vi "WS1050 36 DUT CV Curve Ver1.2.vi"() -> ()   [LabVIEW 2012]
uses:
  WS_VCAP Driver 029/Source/WSVCAP Shell/Type Defs/WSVCAP SHL I2C DUT Mask Mode Enum.ctl
panel:
  out "VISA resource name out":refnum<visa-resource-name>="GPIB0::3::INSTR"
  out "error out 2":errorcluster={"status"=TRUE, "code"=-63192, "source"="niLvFpga_Open_PXI-7813R.vi"}
  in  "Reg1_Bit Cntrl":string[](array[string])=["01", "02", "04", "08", "10", "20", "40", "80", "03", "06", "0C", "D8", "33", "66", "CC", "07", "0E", "1C", "38", "70", "E0", "0F", "1E", "3C", "78", "F0", "1F", "3E", "7C", "F8", "3F", "7E", "FC", "7F", "FE", "FD", "FB", "F7", "EF", "DF", "BF", "7F", "FC", "F9", "F3", "E7", "CF", "9F", "3F", "F8", "F1", "E3", "C7", "8F", "1F", "F0", "E1", "C3", "87", "0F", "E0", "C1", "83", "07", "C0", "81", "03", "AA", "55", "00"]
  out "date string":string="5/19/2014"
  out "PS1 Out":refnum<visa-resource-name>
  out "Ke2000 Out":refnum<visa-resource-name>="GPIB0::9::INSTR"
  in  "Tab Control":T1(tab)
  in  "Board#":string="BRD5"
  in  "Serial Number":string[][](table)=[["DUT", "SN"], ["DUT1", "1"], ["DUT2", "2"], ["DUT3", "3"], ["DUT4", "4"], ["DUT5", "5"], ["DUT6", "6"], ["DUT7", "7"], ["DUT8", "8"], ["DUT9", "9"], ["DUT10", "10"], ["DUT11", "11"], ["DUT12", "12"], ["DUT13", "13"], ["DUT14", "14"], ["DUT15", "15"], ["DUT16", "16"], ["DUT17", "17"], ["DUT18", "18"], ["DUT19", "19"], ["DUT20", "20"], ["DUT21", "21"], ["DUT22", "22"], ["DUT23", "23"], ["DUT24", "24"], ["DUT25", "25"], ["DUT26", "26"], ["DUT27", "27"], ["DUT28", "28"], ["DUT29", "29"], ["DUT30", "30"], ["DUT31", "31"], ["DUT32", "32"], ["DUT33", "33"], ["DUT34", "34"], ["DUT35", "35"], ["DUT36", "36"]]
  in  "Wafer#":string="T7-EB"
  in  "File Name":string="CP Sweep_WS1050_T7_EB_25C_BRD4_160706_1"
  in  "TMN DC\\CAP Data Log File Path":path=path "C:/WS1050 36 DUT Data"
  in  "Test Program":string="WS1050 36 DUT CV Curve Ver1.2"
  out "Current Date":string="8/28/2014"
  out "Current Time":string="0950"
  in  "Start Date":string="10/21/2014"
  in  "Start Time":string="1542"
  in  "Comment":string="CP Sweep RT"
  in  "OK Button":bool
  in  "Calibration":bool
  in  "Verify CP":bool
  in  "CP Setting":i32(ring) items=["CP OFF", "CP ON", "CP 35V", "CP 40V", "DVA ON", "DVA OFF", "REG1 ON", "REG1 OFF", "REG2 ON", "REG2 OFF", "REG3 ON", "REG3 OFF"]
  in  "Set VDD":dbl=3.3 format="%.3g"
  in  "Clock Rate (Hz)":dbl=1000000.0 caption="Meas Speed" format="%.1p Hz"
  out "AR  Measurent(Hz)":dbl
  in  "PS1 Source":refnum<visa-resource-name>="GPIB0::5::INSTR"
  in  "Ke2000":refnum<visa-resource-name>="GPIB0::9::INSTR"
  in  "CP to HD/Cycle":i32(ring)=1 items=["CP HDC 35V", "CP HDC 40.25V", "CP HDC 27.5V", "CP HDC 30.5V", "CP HDC 44V"]
  out "Simulate FPGA":bool
  out "Online":bool
  in  "Ke2400":refnum<visa-resource-name>="GPIB0::3::INSTR"
  in  "Initialize AD7747":bool
  in  "DUT Mask Mode":T2=enum."All"
  in  "RFFE Slave Address":u8=7 caption="Slave Address" format="0x%02x"
  out "Activity Log":string="05/19/2014 -- 12:24:35.853::WSVCAP::APP::Application Started\n05/19/2014 -- 12:24:37.606::WSVCAP::WSVCAP SHL::WR I2C-REG:0x0A;MASK:0xFFFFFFFFFFFF;C1 DATA:22:22:22:22:22:22:22:22:22:22:22:22:22:22:22:22;C2 DATA:22:22:22:22:22:22:22:22:22:22:22:22:22:22:22:22;C3 DATA:22:22:22:22:22:22:22:22:22:22:22:22:22:22:22:22\r\n05/19/2014 -- 12:24:37.773::WSVCAP::WSVCAP SHL::WR I2C-ST:0,0,4,1\r\n05/19/2014 -- 12:24:37.903::WSVCAP::WSVCAP SHL::RD I2C-BYTES:4;ADD:0x00;MASK:0xFFFFFFFFFFFF\r\n05/19/2014 -- 12:24:38.045::WSVCAP::WSVCAP SHL::RD I2C:C1 DATA:2:2:2:2:2:2:2:2:2:2:2:2:2:2:2:2|A7:A9:AA:82:82:7F:82:81:82:81:83:82:81:82:82:81|46:36:BB:88:44:A3:E9:2B:32:20:ED:25:BB:3D:68:B|2C:6A:EB:A7:22:56:FE:CC:36:82:D7:B0:3B:48:F9:CC;C2 DATA:2:2:2:2:2:2:2:2:2:2:2:2:2:2:2:2|94:94:94:80:80:80:80:80:81:7E:7E:81:80:7E:80:80|47:33:15:82:62:B:E8:1C:D7:C3:7D:41:7C:B7:4C:2A|C4:B4:AE:8:1E:D1:4E:37:11:C0:6F:63:42:9D:63:B5;C3 DATA:2:2:2:2:2:2:2:2:2:2:2:2:2:2:2:2|95:95:95:81:81:7E:81:80:84:7D:80:83:81:7E:7F:80|AB:C4:14:B5:7B:52:DF:C9:79:5D:5F:30:99:31:1E:F4|6E:5C:F7:A8:C3:EB:7B:EF:33:92:89:77:4D:67:75:DD;STATUS:0:0:4:0\r\n05/19/2014 -- 12:24:38.046::WSVCAP::WSVCAP SHL::WR I2C-REG:0x0A;MASK:0xFFFFFFFFFFFF;C1 DATA:22:22:22:22:22:22:22:22:22:22:22:22:22:22:22:22;C2 DATA:22:22:22:22:22:22:22:22:22:22:22:22:22:22:22:22;C3 DATA:22:22:22:22:22:22:22:22:22:22:22:22:22:22:22:22\r\n05/19/2014 -- 12:24:38.089::WSVCAP::WSVCAP SHL::WR I2C-ST:0,0,4,1\r\n05/19/2014 -- 12:24:38.219::WSVCAP::WSVCAP SHL::RD I2C-BYTES:4;ADD:0x00;MASK:0xFFFFFFFFFFFF\r\n05/19/2014 -- 12:24:38.362::WSVCAP::WSVCAP SHL::RD I2C:C1 DATA:2:2:2:2:2:2:2:2:2:2:2:2:2:2:2:2|A7:AB:AA:82:82:82:83:83:82:82:82:82:7F:82:82:81|4B:32:96:83:3E:61:43:17:25:62:AB:4D:A2:40:2E:5|3C:76:2B:B4:EE:E4:A9:1A:AA:A:26:C7:21:2E:87:5B;C2 DATA:2:2:2:2:2:2:2:2:2:2:2:2:2:2:2:2|94:94:94:80:80:80:80:80:80:7F:80:81:80:80:7F:80|4A:32:19:7D:19:6C:79:46:61:7F:4B:B8:A5:30:F3:14|B4:70:A:8C:9C:DC:43:FA:1E:A:C6:21:A:A9:13:F3;C3 DATA:2:2:2:2:2:2:2:2:2:2:2:2:2:2:2:2|95:97:94:81:80:81:82:81:80:7E:81:84:7F:81:80:80|B2:32:D0:A7:9E:4C:AB:D4:EE:D9:F0:82:B7:91:7:FF|C1:91:B6:3D:D8:E:1B:4F:9F:6A:F1:6C:E7:3F:7:BA;STATUS:0:0:4:0\r\n05/19/2014 -- 12:24:38.364::WSVCAP::WSVCAP SHL::WR I2C-REG:0x0A;MASK:0xFFFFFFFFFFFF;C1 DATA:22:22:22:22:22:22:22:22:22:22:22:22:22:22:22:22;C2 DATA:22:22:22:22:22:22:22:22:22:22:22:22:22:22:22:22;C3 DATA:22:22:22:22:22:22:22:22:22:22:22:22:22:22:22:22\r\n05/19/2014 -- 12:24:38.406::WSVCAP::WSVCAP SHL::WR I2C-ST:0,0,4,1\r\n05/19/2014 -- 12:24:38.536::WSVCAP::WSVCAP SHL::RD I2C-BYTES:4;ADD:0x00;MASK:0xFFFFFFFFFFFF\r\n05/19/2014 -- 12:24:38.678::WSVCAP::WSVCAP SHL::RD I2C:C1 DATA:2:2:2:2:2:2:2:2:2:2:2:2:2:2:2:2|A7:A9:AB:82:82:81:82:82:82:82:82:82:82:82:82:81|46:71:4C:87:43:3D:7F:FC:25:4F:8E:54:97:3E:60:8C|AA:F4:1F:B5:CE:43:1F:36:9:87:9C:78:86:5:B6:8E;C2 DATA:2:2:2:2:2:2:2:2:2:2:2:2:2:2:2:2|94:94:94:80:7F:7F:80:80:80:80:80:81:80:80:80:80|49:36:18:7D:6E:C5:E4:3C:81:2E:41:D3:75:71:E3:72|E8:D3:E6:D1:E0:48:AE:D4:54:D:E8:8E:B4:41:68:4;C3 DATA:2:2:2:2:2:2:2:2:2:2:2:2:2:2:2:2|95:95:95:81:7F:7F:81:81:81:81:81:84:81:81:82:81|B3:F5:90:AB:82:69:7B:93:D0:77:E8:D5:E8:8C:84:E8|B9:AC:EE:2B:B6:71:8F:4A:74:31:56:BB:8A:B7:A0:C8;STATUS:0:0:4:0\r\n05/19/2014 -- 12:24:38.681::WSVCAP::WSVCAP SHL::WR I2C-REG:0x0A;MASK:0xFFFFFFFFFFFF;C1 DATA:22:22:22:22:22:22:22:22:22:22:22:22:22:22:22:22;C2 DATA:22:22:22:22:22:22:22:22:22:22:22:22:22:22:22:22;C3 DATA:22:22:22:22:22:22:22:22:22:22:22:22:22:22:22:22\r\n05/19/2014 -- 12:24:38.723::WSVCAP::WSVCAP SHL::WR I2C-ST:0,0,4,1\r\n05/19/2014 -- 12:24:38.854::WSVCAP::WSVCAP SHL::RD I2C-BYTES:4;ADD:0x00;MASK:0xFFFFFFFFFFFF\r\n05/19/2014 -- 12:24:38.996::WSVCAP::WSVCAP SHL::RD I2C:C1 DATA:2:2:2:2:2:2:2:2:2:2:2:2:2:2:2:2|A7:A9:AA:82:82:7F:83:81:82:81:84:82:7F:82:7F:82|43:FB:E:7F:3C:AD:35:35:26:A2:6C:21:4B:3D:8:6|63:9A:E1:F3:95:32:91:42:90:3C:78:1F:5C:D7:5F:D8;C2 DATA:2:2:2:2:2:2:2:2:2:2:2:2:2:2:2:2|94:94:94:80:80:80:80:80:81:80:7E:81:80:7E:7F:80|48:36:18:7F:5E:3D:69:83:DE:AE:A1:9E:31:AE:BB:96|15:A0:44:17:13:FD:CC:C8:6D:B2:EF:A7:C:C7:3B:F;C3 DATA:2:2:2:2:2:2:2:2:2:2:2:2:2:2:2:2|95:96:94:81:81:7E:82:80:84:80:80:84:7F:7E:7D:82|AD:3B:6D:A9:7C:57:9D:F5:7A:96:23:5C:36:2D:ED:5A|CD:46:DB:3B:C7:BD:70:60:33:B8:B:F7:63:A:51:4D;STATUS:0:0:4:0\r\n05/19/2014 -- 12:24:38.998::WSVCAP::WSVCAP SHL::WR I2C-REG:0x0A;MASK:0xFFFFFFFFFFFF;C1 DATA:22:22:22:22:22:22:22:22:22:22:22:22:22:22:22:22;C2 DATA:22:22:22:22:22:22:22:22:22:22:22:22:22:22:22:22;C3 DATA:22:22:22:22:22:22:22:22:22:22:22:22:22:22:22:22\r\n05/19/2014 -- 12:24:39.040::WSVCAP::WSVCAP SHL::WR I2C-ST:0,0,4,1\r\n05/19/2014 -- 12:24:39.170::WSVCAP::WSVCAP SHL::RD I2C-BYTES:4;ADD:0x00;MASK:0xFFFFFFFFFFFF\r\n05/19/2014 -- 12:24:39.311::WSVCAP::WSVCAP SHL::RD I2C:C1 DATA:2:2:2:2:2:2:2:2:2:2:2:2:2:2:2:2|A7:AA:AB:82:82:81:82:81:82:81:82:82:82:82:7F:82|44:F1:90:87:45:44:C8:2C:2C:F1:FC:1B:94:3B:3C:75|4A:49:95:19:99:73:64:3:23:24:F3:A2:5E:7F:C4:B6;C2 DATA:2:2:2:2:2:2:2:2:2:2:2:2:2:2:2:2|94:94:94:80:80:80:80:7F:80:80:7E:80:80:7E:7F:80|4C:36:17:7D:A8:9F:DE:C7:53:6D:8A:F4:41:A5:C6:E0|90:2E:24:C:D9:22:E4:76:3B:40:1D:53:33:B1:3E:4D;C3 DATA:2:2:2:2:2:2:2:2:2:2:2:2:2:2:2:2|95:97:95:81:81:7F:81:80:80:81:7F:82:81:7E:7D:82|AE:2B:A7:AB:CC:CD:A4:38:FD:17:80:F2:92:2D:45:C4|76:E5:D:B9:AD:B5:BA:8D:28:32:9E:42:B7:20:4A:D9;STATUS:0:0:4:0\r\n05/19/2014 -- 12:24:39.313::WSVCAP::WSVCAP SHL::WR I2C-REG:0x0A;MASK:0xFFFFFFFFFFFF;C1 DATA:22:22:22:22:22:22:22:22:22:22:22:22:22:22:22:22;C2 DATA:22:22:22:22:22:22:22:22:22:22:22:22:22:22:22:22;C3 DATA:22:22:22:22:22:22:22:22:22:22:22:22:22:22:22:22\r\n05/19/2014 -- 12:24:39.355::WSVCAP::WSVCAP SHL::WR I2C-ST:0,0,4,1\r\n05/19/2014 -- 12:24:39.486::WSVCAP::WSVCAP SHL::RD I2C-BYTES:4;ADD:0x00;MASK:0xFFFFFFFFFFFF\r\n05/19/2014 -- 12:24:39.628::WSVCAP::WSVCAP SHL::RD I2C:C1 DATA:2:2:2:2:2:2:2:2:2:2:2:2:2:2:2:2|A7:A9:AA:82:82:82:83:82:82:82:82:82:7F:82:7F:82|47:18:E4:87:3E:E7:6:65:25:92:37:38:A8:3E:89:85|7C:A7:7:2B:A3:7A:EC:EF:89:ED:F4:D3:D8:BC:3A:F5;C2 DATA:2:2:2:2:2:2:2:2:2:2:2:2:2:2:2:2|94:94:94:80:7F:80:80:7F:81:80:7E:80:80:80:81:80|49:37:17:80:76:25:6A:F8:DF:55:97:4D:B8:5B:2B:B1|13:E3:9A:3E:1A:2D:4F:B6:DB:E9:61:FA:8B:D6:9:CC;C3 DATA:2:2:2:2:2:2:2:2:2:2:2:2:2:2:2:2|95:95:95:81:7F:80:82:81:84:80:7F:81:80:81:7F:82|AF:93:3B:AF:5B:11:82:E4:7E:C3:2D:72:9:96:D9:A|DB:96:F2:10:5F:64:9A:C6:98:12:27:7D:10:D3:20:D9;STATUS:0:0:4:0\r\n05/19/2014 -- 12:24:40.132::WSVCAP::WSVCAP SHL::CLOSE\r\n"
  in  "C1 Cap DAC":u8=128 caption="B Data In" format="0x%02x"
  in  "C2 Cap DAC":u8=128 caption="B Data In" format="0x%02x"
  in  "C3 Cap DAC":u8=128 caption="B Data In" format="0x%02x"
  out "IDD Brd(uA)":string
  in  "Control Panel":T3={"Verify Socket"=FALSE, "HD/CYC"=FALSE, "E-CAL"=FALSE, "DVA"=FALSE, "VPI"=TRUE, "VSA"=FALSE, "HS"=FALSE}
  out "Verify Socket":bool
  out "HD/CYC":bool
  out "E-CAL":bool
  out "DVA":bool
  out "VPI":bool
  out "VSA":bool
  out "HS":bool
  in  "Lot#":string="WS1050"
  out "AD7747 Values":string[][](table)
  in  "Freq(Hz)":string="NA"
  in  "Reset P/S":bool
  in  "Test Sequences":i32(ring) items=["C1_C2_C3", "C2_C1_C3", "C3_C2_C1"]
  in  "WS1050/51":bool=TRUE
  in  "CP with DVA ON":i32(ring) items=["CP HDC 35V", "CP HDC 40.25V", "CP HDC 27.5V", "CP HDC 30.5V", "CP HDC 44V"]
  in  "CP Sweep":bool=TRUE
  in  "Serialize":bool
  in  "Start No":i32=1
  in  "VPI Name":string[](array[string])=["All Drivers ON"]
  in  "VPI_Cmd":string[](array[string])=["3B"]
  in  "Temperature":string="25C"
  out "40V_1":string[][](table)
  out "NOM IDD OFF(uA)":string
  out "40V_2":string[][](table)
  out "40V_3":string[][](table)
  out "Previous Time":string="12:20:26 PM"
  out "STATUS":string="Idle...."
  out "Total Delta C2(pF)":string[](array[string])
  out "Total Delta C1(pF)":string[](array[string])
  out "Total Delta C3(pF)":string[](array[string])
  out "RB Reg for HD/Cycle":string[](array[string])
  out "VPI C2":string[][](table)
  out "VPI C3":string[][](table)
  out "NOM IDD ON (uA)":string
  out "IDD_HD/CYC (uA)":string="164.601255E+0"
  in  "stop":bool
  out "IDD Stdby(uA)":string="2.606990E+0"
  out "VPI C1":string[][](table)
  in  "TTF Completed":i32=60
  out "Loop Completed":i32
  out "VSA_V1":string[][](table)
  out "VSA_V2":string[][](table)
  out "VSA_V3":string[][](table)
  in  "VSA Voltage(V)":dbl[](array[numeric])=[-27.0, 0.0, 27.0]
  in  "X Repeat":i32=100
  out "% Delta C_T0":string[][](array[string])
  out "% Delta C":string[][](array[string])
  out "EFuse RB T0":string[](array[string])
  out "Current EFuse Read back":string[](array[string])
  out "EFuse Readback Status":bool[](array[boolean])
  in  "DeltaC Target Setting(pF)":dbl=7.375
  out "error out":errorcluster
  in  "error in (no error)":errorcluster
  in  "Bank 2":i32(ring)=1 items=["C1", "C2", "C3", "D_C1", "D_C2", "D_C3"]
  out "DeltaC Change_1":dbl[][](graph) caption="(Y) Multi Plot 2"
  out "DeltaC Change_2":dbl[][](graph) caption="(Y) Multi Plot 2"
  out "DeltaC Change_3":dbl[][](graph) caption="(Y) Multi Plot 2"
  in  "Debug":bool
  in  "No of Rows\nFrom Spread Sheet":i32
  in  "Plot Delta Cmin":bool=TRUE
  in  "Plot":T4(ring)
  in  "Bank 1":i32(ring) items=["C1", "C2", "C3", "D_C1", "D_C2", "D_C3"]
  in  "Bank 3":i32(ring)=2 items=["C1", "C2", "C3", "D_C1", "D_C2", "D_C3"]
  in  "Col C1":i32=5
  in  "Col C2":i32=6
  in  "Col C3":i32=7
  # "Company:  WiSpry Inc\n20 Fairbanks Ste 198 Irvine CA 92618\n\nAuthor:  Andy V Tran\nCreated:  07/06/2016\nLabVIEW 2012 Pro\nTest Program:  WS1050 36 DUT \nCP Sweep ver1.2\nFPGA: WS_VCAP Driver 029"
  # "Note for CP CV Sweep:\n\n1.  CP will sweep from Low to High to Low\n2.  CP will sweep by banks\n3.  VPI will be checked for CP CV Sweep"
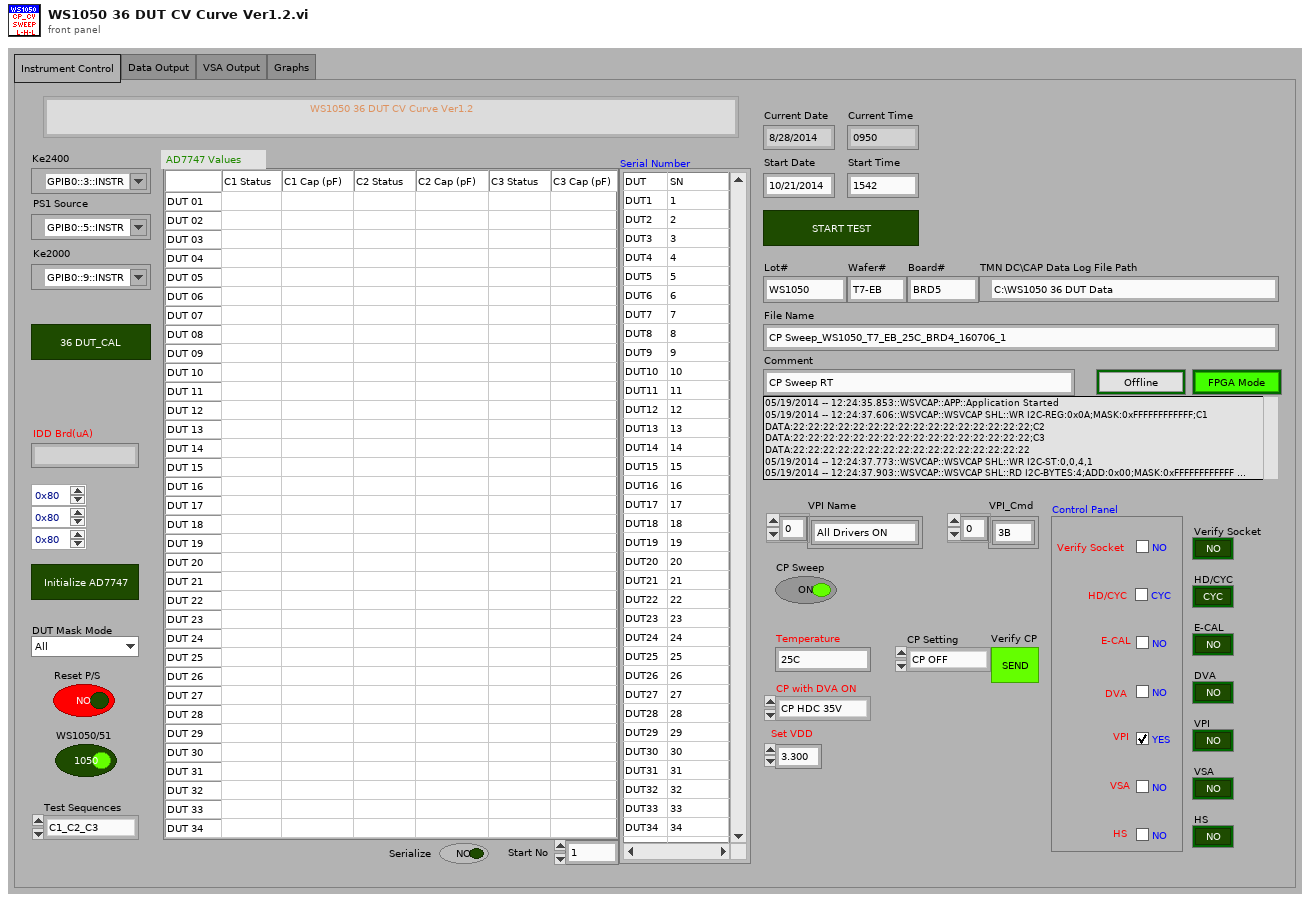
[diagram p1: front panel]
types:
  T1 = enum32{"Instrument Control", "Data Output", "VSA Output", "Graphs"}
  T2 = typedef "WSVCAP SHL I2C DUT Mask Mode Enum.ctl" = enum16{"Custom", "C1", "C2", "C3", "All"}
  T3 = cluster{"Verify Socket":bool, "HD/CYC":bool, "E-CAL":bool, "DVA":bool, "VPI":bool, "VSA":bool, "HS":bool}
  T4 = enum16{"ALL DUTs", "DUT 01", "DUT 02", "DUT 03", "DUT 04", "DUT 05", "DUT 06", "DUT 07", "DUT 08", "DUT 09", "DUT 10", "DUT 11", "DUT 12", "DUT 13", "DUT 14", "DUT 15", "DUT 16", "DUT 17", "DUT 18", "DUT 19", "DUT 20", "DUT 21", "DUT 22", "DUT 23", "DUT 24", "DUT 25", "DUT 26", "DUT 27", "DUT 28", "DUT 29", "DUT 30", "DUT 31", "DUT 32", "DUT 33", "DUT 34", "DUT 35", "DUT 36"}
  T5 = typedef "WSVCAP SHL Core System Cluster.ctl" = cluster{"Settings":T6, "FPGA Resource":tag, "Online":bool, "I2C Wait Ticks":u32, "SPI Wait Ticks":u32, "RFFE Wait Ticks":u32}
  T6 = typedef "WSVCAP SHL I2C Settings Cluster.ctl" = cluster{"FPGA Resource Name":string, "I2C Slave Address":u8, "I2C Clock Rate (Hz)":dbl, "SPI Clock Rate (Hz)":dbl, "RFFE Slave Address":u8, "RFFE Clock Rate (Hz)":dbl, "Simulate FPGA":bool, "C1 Cap DAC Default":u8, "C2 Cap DAC Default":u8, "C3 Cap DAC Default":u8}
  T7 = enum16{"Idle...", "Voltage 1", "Voltage 2", "Voltage 3"}
  T8 = enum16{"Idle...", "Voltage 1", "Voltage 2", "Voltage 3"}[]
  T9 = cluster{"Test Program ":string, "Comment":string, "Data Out":string, "Data Out":string, "Data Out":string, string, "Data Out":string, "Data Out":string, "Data Out":string, "Freq(Hz)":string, "Board#":string}
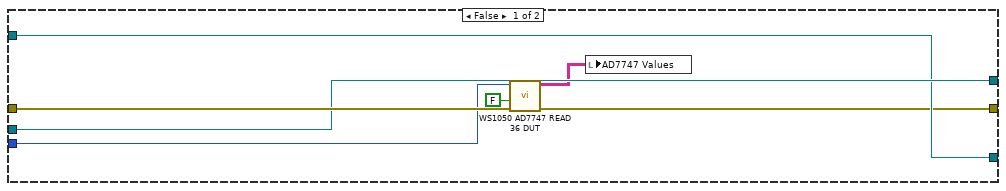
[diagram p9: hidden frame]
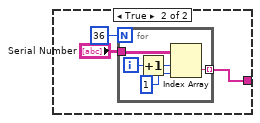
[diagram p10: hidden frame]
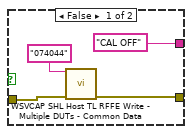
[diagram p11: hidden frame]
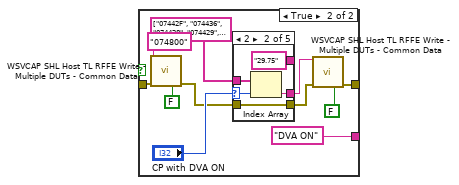
[diagram p12: hidden frame]
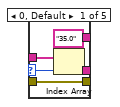
[diagram p13: hidden frame]
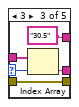
[diagram p14: hidden frame]
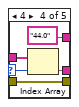
[diagram p15: hidden frame]
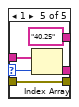
[diagram p16: hidden frame]
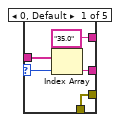
[diagram p17: hidden frame]
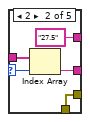
[diagram p18: hidden frame]
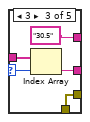
[diagram p19: hidden frame]
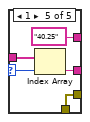
[diagram p20: hidden frame]
diagram:
  w18 = TRUE
  w24 = u16 0 items=["Off", "Moving Filter", "Repeating Filter"] ("Digital Filter (0: Off)")
  w25 = u16 7 items=["3.5 Digits"=4, "4.5 Digits"=5, "5.5 Digits"=6, "6.5 Digits"=7] ("Resolution (7: 6.5 digits)")
  n1 = case shown="True" w18 {
    tunnel: "error in (no error)" -> [w31 w32]
    tunnel: [w31 w39] -> w5
    frame False {
    }
    frame True {
      n2 = call "WSVCAP SHL Host TL Initialize.vi"("error in"=w32) -> ("error out"=w33:errorcluster)  [unwired: 13 in, 1 out]
      n3 = control-ref of="Activity Log"() -> (w35:refnum<vi>)
      n4 = call "ACT LG Activity Log Core.vi"("Display Ref"=w35, "Source"="WSVCAP", "Error In (no error)"=w33) -> ("Error Out"=w34:errorcluster)  [unwired: 11 in, 1 out]
      n5 = call "WSVCAP SHL Host TL Status Manager.vi"("error in"=w34) -> ("System Out"=w40:T5, "error out"=w39:errorcluster)  [unwired: 13 in]
      n6 = Unbundle By Name(w40) -> ("Online"=→"Online":bool, "Settings.Simulate FPGA"=→"Simulate FPGA":bool)
    }
  }
  n7 = case shown="True" TRUE {
    tunnel: w5 -> [w41 w46]
    tunnel: [w42 w45] -> w15
    tunnel: [w41 w44] -> w9
    tunnel: "Ke2400" -> [w42 w43]
    frame False {
    }
    frame True {
      n8 = VISA Write(VISA resource name=w43, write buffer="SOUR:FUNC VOLT;VOLT:MODE FIX;RANG 100;LEV 0.0;:SENS:FUNC \"CURR\";CURR:PROT 60E-3;RANG 100E-3;:OUTP ON", error in (no error)=w46) -> (VISA resource name out=w45:refnum<visa-resource-name>, error out=w44:errorcluster)  [unwired: 1 out]
    }
  }
  n9 = case shown="True" "Reset P/S" {
    tunnel: "PS1 Source" -> [w48 w55]
    tunnel: [w48 w53] -> w29
    tunnel: w5 -> [w49 w51]
    tunnel: [w49 w50] -> w4
    frame False {
    }
    frame True {
      n10 = call "Agilent 3631A Initialize.vi"("error in (no error)"=w51, "Default"=FALSE ("Reset? (T: Yes)"), "Reset"=TRUE ("ID Query? (T: Yes)"), "VISA resource name"=w55) -> ("error out"=w50:errorcluster, "VISA resource name out"=w53:refnum<visa-resource-name>)  [unwired: 6 in]
    }
  }
  n11 = call "Ke2000 Initialize.vi"("error in (no error)"=w5, "VISA resource name"="Ke2000") -> ("error out"=w26:errorcluster, "VISA resource name out"=w27:refnum<visa-resource-name>)  [unwired: 8 in]
  n12 = call "Ke2000 Configure DC Current.vi"("Resolution (7: 6.5 digits)"=w25, "Digital Filter (0: Off)"=w24, "Auto Range? (T: Auto)"=FALSE, "error in"=w26, "Custom Range (0 A)"=1.0, "VISA resource name"=w27) -> ("error out"=w6:errorcluster, "VISA resource name out"=w22:refnum<visa-resource-name>)  [unwired: 4 in]
  n13 = Merge Errors(w9, w6, w4) -> (w16:errorcluster)
  n14 = while {
    tunnel: w16 -> [w61]
    tunnel: [w64] -> w12
    tunnel: w29 -> [w68]
    tunnel: w22 -> [w69]
    tunnel: [w78] -> w21
    tunnel: [w77] -> w20
    tunnel: w15 -> [w75]
    tunnel: [w74] -> w13
    tunnel: [FALSE ("stop")] -> w7
    i -> [w76]
    stop <- w80 stop-if-true
    n15 = case shown="0" w76 {
      tunnel: w61 -> [w91 w92]
      tunnel: [w90 w92] -> w71
      tunnel: "RFFE Slave Address" -> [w88 _]
      frame 0 {
        w84 = dbl[][] []
        w83 = "" ("uA")
        w85 = string[][] []
        w86 = string[] [] ("EFuse Read back")
        n16 = local write "RB Reg for HD/Cycle"(w86) -> ()
        n17 = local write "Current EFuse Read back"(w86) -> ()
        n18 = local write "EFuse RB T0"(w86) -> ()
        n19 = local write "Total Delta C1(pF)"(w86) -> ()
        n20 = local write "Total Delta C2(pF)"(w86) -> ()
        n21 = local write "Total Delta C3(pF)"(w86) -> ()
        n22 = local write "VPI C2"(w85) -> ()
        n23 = local write "VSA_V3"(w85) -> ()
        n24 = local write "VSA_V1"(w85) -> ()
        n25 = local write "40V_2"(w85) -> ()
        n26 = local write "40V_1"(w85) -> ()
        n27 = local write "NOM IDD OFF(uA)"(w83) -> ()
        n28 = local write "NOM IDD ON (uA)"(w83) -> ()
        n29 = local write "IDD Brd(uA)"(w83) -> ()
        n30 = local write "VSA_V2"(w85) -> ()
        n31 = local write "VPI C1"(w85) -> ()
        n32 = local write "VPI C3"(w85) -> ()
        n33 = local write "% Delta C"(w85) -> ()
        n34 = local write "% Delta C_T0"(w85) -> ()
        n35 = local write "40V_3"(w85) -> ()
        n36 = call "WSVCAP SHL Host TL RFFE Configure.vi"("RFFE Slave Address"=w88, "Clock Rate (Hz)"="Clock Rate (Hz)", "error in"=w91) -> ("Actual Rate (Hz)"=→"AR  Measurent(Hz)":dbl, "error out"=w90:errorcluster)  [unwired: 11 in]
        n37 = local write "DeltaC Change_3"(w84) -> ()
        n38 = local write "DeltaC Change_1"(w84) -> ()
        n39 = local write "DeltaC Change_2"(w84) -> ()
      }
      frame 1, Default {
      }
    }
    n40 = while {
      tunnel: ["stop"] -> w73
      tunnel: w71 -> [w113]
      tunnel: [w105] -> w65
      tunnel: w68 -> [w112]
      tunnel: w69 -> [w107]
      tunnel: [w108] -> w67
      tunnel: [w106] -> w66
      tunnel: [w103] -> w63
      tunnel: [w102] -> w62
      tunnel: [w101] -> w60
      tunnel: [w100] -> w59
      tunnel: [w99] -> w58
      tunnel: [w98] -> w57
      tunnel: [w97] -> w56
      stop <- w120 stop-if-true
      # "Set Date & Time to Start Test"
      n41 = case shown="True" "Initialize AD7747" {
        tunnel: w113 -> [w129 w134]
        tunnel: [w129 w130] -> w96
        tunnel: w112 -> [w128 w132]
        tunnel: [w128 w131] -> w111
        frame False {
        }
        frame True {
          w135 = T8 [enum."Voltage 2", enum."Voltage 3", enum."Voltage 1"] items=["Idle...", "Voltage 1", "Voltage 2", "Voltage 3"]
          n42 = for {
            tunnel: w132 -> [w145]
            tunnel: w135 -> [w143] mode=indexing
            tunnel: [w142] -> w131
            shift-right: [w138] -> w133
            shift-left: w134 -> [w146]
            n43 = local read "Set VDD"() -> (w141:dbl)
            n44 = call "E3631A_Voltage Controller updated.vi"("VISA resource name"=w145, "I_VDD(A)"=0.5, "Channel Controller"=w143, "Voltage 1"=w141, "Voltage 2"=3.3, "error in (no error)"=w146, "I_3.3V (A)"=0.5) -> ("VISA resource name out"=w142:refnum<visa-resource-name>, "error out"=w137:errorcluster)  [unwired: 7 in]
            n45 = call "Delay.vi"("milliseconds to wait"=u32 100, "error in (no error)"=w137) -> ("error out"=w138:errorcluster)  [unwired: 9 in]
          }
          n46 = call "WS1050_AD7747_Init 36DUT.vi"("error in"=w133) -> ("error out"=w130:errorcluster)  [unwired: 10 in]
        }
      }
      n47 = call "Time_stamp.vi"() -> ("date/time string"=w125:string, "date string"=w127:string)  [unwired: 2 in]
      "Current Date" <- w127
      "Current Time" <- w125
      n48 = Equal?(x=w127, y="Start Date") -> (x = y?=w123:bool)
      n49 = Equal?(x=w125, y="Start Time") -> (x = y?=w122:bool)
      n50 = And(x=w123, y=w122) -> (x .and. y?=w119:bool)
      n51 = Compound Arithmetic op=OR(w119, "OK Button", "stop") -> (w120:bool)
      n52 = case shown="True" "Calibration" {
        tunnel: w96 -> [w176 w193]
        tunnel: [w170 w190] -> w94
        tunnel: w111 -> [w175 w189]
        tunnel: "DUT Mask Mode" -> [w174 w185]
        tunnel: [w175 w184] -> w109
        tunnel: w107 -> [w173 w180]
        tunnel: [w173 w177] -> w106
        frame False {
          n53 = call "WS1050 AD7747 READ 36 DUT.vi"("error in"=w176, "Log (T)"=FALSE, "DUT Mask Mode (All)"=w174) -> ("error out"=w170:errorcluster, "AD7747 Values"=w171:string[][])  [unwired: 7 in]
          n54 = local write "AD7747 Values"(w171) -> ()
        }
        frame True {
          n55 = flat-sequence {
            tunnel: w193 -> [w207]
            tunnel: [w202] -> w192
            tunnel: w189 -> [w206]
            tunnel: [w205] -> w188
            tunnel: w185 -> [w204]
            tunnel: [w204] -> w186
            tunnel: w180 -> [w200]
            tunnel: [w199] -> w179
            tunnel: w192 -> [w221]
            tunnel: [w220] -> w191
            tunnel: w188 -> [w219]
            tunnel: [w219] -> w187
            tunnel: w186 -> [w218]
            tunnel: "C1 Cap DAC" -> [w214]
            tunnel: "C2 Cap DAC" -> [w213]
            tunnel: "C3 Cap DAC" -> [w212]
            tunnel: w179 -> [w211]
            tunnel: [w211] -> w178
            tunnel: w191 -> [w229]
            tunnel: [w231] -> w190
            tunnel: w187 -> [w230]
            tunnel: [w228] -> w184
            tunnel: w178 -> [w227]
            tunnel: [w227] -> w177
            frame #0 {
              w194 = 0.5 ("I_VDD(A)")
              n56 = local read "Set VDD"() -> (w196:dbl)
              n57 = call "E3631A_Voltage Controller updated.vi"("VISA resource name"=w206, "I_VDD(A)"=w194, "Channel Controller"=T7."Voltage 1", "Voltage 1"=w196, "error in (no error)"=w207, "I_3.3V (A)"=w194) -> ("VISA resource name out"=w205:refnum<visa-resource-name>, "error out"=w197:errorcluster)  [unwired: 8 in]
              n58 = call "Delay.vi"("milliseconds to wait"=u32 100, "error in (no error)"=w197) -> ("error out"=w201:errorcluster)  [unwired: 9 in]
              n59 = call "Ke2000 Single Reading.vi"("error in (no error)"=w201, "VISA resource name"=w200) -> ("error out"=w202:errorcluster, "VISA resource name out"=w199:refnum<visa-resource-name>, "uA"=→"IDD Brd(uA)":string)  [unwired: 5 in, 2 out]
              n60 = One Button Dialog(message="Please verify all sockets should be empty...") -> ()  [unwired: 1 in, 1 out]
            }
            frame #1 {
              n61 = call "WS1050 CAPDAC Setting.vi"("DUT Mask Mode (All)"=w218, "error in"=w221, "C3 Cap DAC"=w212, "C2 Cap DAC"=w213, "C1 Cap DAC"=w214) -> ("error out"=w216:errorcluster)  [unwired: 6 in]
              n62 = call "WS1050 OFFSET CAL_In Series.vi"("error in"=w216, "OFFSET CAL"=TRUE ("Read?")) -> ("error out"=w215:errorcluster)  [unwired: 9 in]
              n63 = call "WS1050 AD7747 READ 36 DUT.vi"("error in"=w215, "Log (T)"=FALSE, "DUT Mask Mode (All)"=w218) -> ("error out"=w220:errorcluster, "AD7747 Values"=→"AD7747 Values":string[][])  [unwired: 7 in]
            }
            frame #2 {
              w222 = 0.5 ("I_3.3V (A)")
              n64 = call "E3631A_Voltage Controller updated.vi"("VISA resource name"=w230, "I_VDD(A)"=w222, "Channel Controller"=T7."Voltage 1", "Voltage 1"=0.0, "error in (no error)"=w229, "I_3.3V (A)"=w222) -> ("VISA resource name out"=w228:refnum<visa-resource-name>, "error out"=w224:errorcluster)  [unwired: 8 in]
              n65 = call "Delay.vi"("milliseconds to wait"=u32 100, "error in (no error)"=w224) -> ("error out"=w231:errorcluster)  [unwired: 9 in]
              n66 = One Button Dialog(message="Calibration Completed....") -> ()  [unwired: 1 in, 1 out]
            }
          }
        }
      }
      n67 = call "Control Panel.vi"("error in (no error)"=w96, "Control Panel"="Control Panel") -> ("error out"=w93:errorcluster, "VPI"=w99:bool, "DVA"=w100:bool, "E-CAL"=w101:bool, "VSA"=w98:bool, "HD/CYC"=w102:bool, "HS"=w97:bool, "Verify Socket"=w103:bool)  [unwired: 2 in]
      "Verify Socket" <- w103
      "E-CAL" <- w101
      "VPI" <- w99
      "VSA" <- w98
      "HS" <- w97
      "HD/CYC" <- w102
      "DVA" <- w100
      n68 = Merge Errors(w93, w94) -> (w95:errorcluster)
      n69 = case shown="True" "Verify CP" {
        tunnel: [w147 w151] -> w105
        tunnel: w109 -> [w148 w154]
        tunnel: [w148 w152] -> w108
        tunnel: w95 -> [w147 w150]
        frame False {
        }
        frame True {
          w155 = T8 [enum."Voltage 2", enum."Voltage 3", enum."Voltage 1"] items=["Idle...", "Voltage 1", "Voltage 2", "Voltage 3"]
          # "Verify CP"
          n70 = for {
            tunnel: w154 -> [w168]
            tunnel: w155 -> [w166] mode=indexing
            shift-right: [w163] -> w153
            shift-left: w150 -> [w169]
            tunnel: [w161] -> w152
            n71 = local read "Set VDD"() -> (w165:dbl)
            n72 = call "E3631A_Voltage Controller updated.vi"("VISA resource name"=w168, "I_VDD(A)"=0.5, "Channel Controller"=w166, "Voltage 1"=w165, "Voltage 2"=3.3, "error in (no error)"=w169, "I_3.3V (A)"=0.5) -> ("VISA resource name out"=w161:refnum<visa-resource-name>, "error out"=w164:errorcluster)  [unwired: 7 in]
            n73 = call "Delay.vi"("milliseconds to wait"=u32 100, "error in (no error)"=w164) -> ("error out"=w163:errorcluster)  [unwired: 9 in]
          }
          n74 = Index Array(array=string[] ["074000", "074040", "07476F", "074776", "074800", "074820", "07413B", "074100", "07423B", "074200", "07433B", "074300"], index="CP Setting") -> (element=w156:string)
          n75 = call "WSVCAP SHL Host TL RFFE Write - Multiple DUTs - Common Data.vi"("Data Out"=w156, "error in"=w153, "Log (T)"=FALSE) -> ("error out"=w151:errorcluster)  [unwired: 12 in]
        }
      }
      n76 = Wait Until Next ms Multiple(millisecond multiple=u32 100) -> ()  [unwired: 1 out]
    }
    n77 = case shown="False" w73 {
      tunnel: w65 -> [w287 w1529]
      tunnel: [w272 w1529] -> w64
      tunnel: w67 -> [w286 w1527]
      tunnel: w66 -> [w278 w1528]
      tunnel: [w284 w1528] -> w78
      tunnel: [w282 w1527] -> w77
      tunnel: w75 -> [w275 w1526]
      tunnel: [w271 w1526] -> w74
      tunnel: "RFFE Slave Address" -> [w269 _]
      tunnel: [FALSE ("stop During HD/Cycles") FALSE ("stop During HD/Cycles")] -> _
      tunnel: w63 -> [w246 _]
      tunnel: w62 -> [_ _]
      tunnel: w60 -> [w245 _]
      tunnel: w59 -> [w244 _]
      tunnel: w58 -> [w243 _]
      tunnel: w57 -> [w242 _]
      tunnel: w56 -> [w241 _]
      frame False {
        w249 = u32 100 ("milliseconds to wait")
        w283 = T8 [enum."Voltage 2", enum."Voltage 3", enum."Voltage 1"] items=["Idle...", "Voltage 1", "Voltage 2", "Voltage 3"]
        w285 = T8 [enum."Voltage 2", enum."Voltage 3", enum."Voltage 1"] items=["Idle...", "Voltage 1", "Voltage 2", "Voltage 3"]
        n78 = for {
          tunnel: w287 -> [w1524]
          tunnel: w286 -> [w1523]
          tunnel: w285 -> [w1521] mode=indexing
          tunnel: [w1516] -> w280
          tunnel: [w1520] -> w270
          n79 = local read "Set VDD"() -> (w1519:dbl)
          n80 = call "E3631A_Voltage Controller updated.vi"("VISA resource name"=w1523, "I_VDD(A)"=0.5, "Channel Controller"=w1521, "Voltage 1"=w1519, "Voltage 2"=3.3, "error in (no error)"=w1524, "I_3.3V (A)"=0.5) -> ("VISA resource name out"=w1520:refnum<visa-resource-name>, "error out"=w1517:errorcluster)  [unwired: 7 in]
          n81 = call "Delay.vi"("milliseconds to wait"=u32 100, "error in (no error)"=w1517) -> ("error out"=w1516:errorcluster)  [unwired: 9 in]
        }
        n82 = call "WSVCAP SHL Host TL RFFE Write - Multiple DUTs - Common Data.vi"("Data Out"="074000", "error in"=w280, "Log (T)"=FALSE) -> ("error out"=w281:errorcluster)  [unwired: 12 in]
        n83 = local read "IDD Brd(uA)"() -> (w258:string)
        n84 = case shown="False" "Serialize" {
          tunnel: [w289 w299] -> w248
          frame False {
            w288 = 36
            n85 = for {
              N: w288 -> [_]
              tunnel: [w294] -> w290 mode=indexing
              i -> [w298]
              n86 = Add(x="Start No", y=w298) -> (x+y=w296:i32)
              n87 = Number To Fractional String(number=w296, precision (6)=i16 0) -> (F-format string=w294:string)  [unwired: 2 in]
            }
            n88 = for {
              N: w288 -> [_]
              tunnel: w290 -> [w293]
              tunnel: [w292] -> w289 mode=indexing
              i -> [w291]
              n89 = Index Array(array=w293, index=w291) -> (element=w292:string)
            }
          }
          frame True {
            n90 = for {
              N: 36 -> [_]
              tunnel: "Serial Number" -> [w306]
              tunnel: [w304] -> w299 mode=indexing
              i -> [w303]
              n91 = Increment(x=w303) -> (x+1=w302:i32)
              n92 = Index Array(array=w306, index (row)=w302, index (col)=1 ("disabled index (col)")) -> (element=w304:string)
            }
          }
        }
        n93 = call "Delay.vi"("milliseconds to wait"=w249, "error in (no error)"=w281) -> ("error out"=w279:errorcluster)  [unwired: 9 in]
        n94 = call "Ke2000 Single Reading.vi"("error in (no error)"=w279, "VISA resource name"=w278) -> ("error out"=w259:errorcluster, "VISA resource name out"=w277:refnum<visa-resource-name>, "uA"=w261:string)  [unwired: 5 in, 2 out]
        n95 = call "Substration.vi"("error in (no error)"=w259, "Input2"=w258, "Input1"=w261) -> ("error out"=w237:errorcluster, "In1 - In2"=w260:string)  [unwired: 7 in]
        "IDD Stdby(uA)" <- w260
        n96 = call "WSVCAP SHL Host TL RFFE Write - Multiple DUTs - Common Data.vi"("Data Out"="074040", "error in"=w237, "Log (T)"=FALSE) -> ("error out"=w236:errorcluster)  [unwired: 12 in]
        n97 = call "Delay.vi"("milliseconds to wait"=w249, "error in (no error)"=w236) -> ("error out"=w267:errorcluster)  [unwired: 9 in]
        n98 = case shown="False" w244 {
          tunnel: w267 -> [w324 w333]
          tunnel: [w323 w331] -> w265
          tunnel: ["DVA OFF" ("Data Out") "DVA ON" ("Data Out")] -> w266
          frame False {
            n99 = call "WSVCAP SHL Host TL RFFE Write - Multiple DUTs - Common Data.vi"("Data Out"="074820", "error in"=w324) -> ("error out"=w323:errorcluster)  [unwired: 13 in]
          }
          frame True {
            n100 = call "WSVCAP SHL Host TL RFFE Write - Multiple DUTs - Common Data.vi"("Data Out"="074800", "error in"=w333, "Log (T)"=FALSE) -> ("error out"=w329:errorcluster)  [unwired: 12 in]
            n101 = case shown="2" "CP with DVA ON" {
              selector: "CP with DVA ON" -> [w339 w344 w349 w354 w358]
              tunnel: string[] ["07442F", "074436", "074428", "074429", "07443B"] -> [w340 w345 w350 w355 w360]
              tunnel: [w338 w343 w348 w353 w359] -> w325
              tunnel: ["35.0" ("Data Out") "29.75" ("Data Out") "30.5" ("Data Out") "44.0" ("Data Out") "40.25" ("Data Out")] -> _
              tunnel: w329 -> [w336 w341 w346 w351 w356]
              tunnel: [w336 w341 w346 w351 w356] -> w328
              frame 0, Default {
                n102 = Index Array(array=w340, index=w339) -> (element=w338:string)
              }
              frame 2 {
                n103 = Index Array(array=w345, index=w344) -> (element=w343:string)
              }
              frame 3 {
                n104 = Index Array(array=w350, index=w349) -> (element=w348:string)
              }
              frame 4 {
                n105 = Index Array(array=w355, index=w354) -> (element=w353:string)
              }
              frame 1 {
                n106 = Index Array(array=w360, index=w358) -> (element=w359:string)
              }
            }
            n107 = call "WSVCAP SHL Host TL RFFE Write - Multiple DUTs - Common Data.vi"("Data Out"=w325, "error in"=w328, "Log (T)"=FALSE) -> ("error out"=w331:errorcluster)  [unwired: 12 in]
          }
        }
        n108 = Not(x=w241) -> (.not. x?=w247:bool)
        n109 = Number To Fractional String(number="Set VDD", precision (6)=i16 2) -> (F-format string=w263:string)  [unwired: 2 in]
        n110 = call "Delay.vi"("milliseconds to wait"=w249, "error in (no error)"=w265) -> ("error out"=w253:errorcluster)  [unwired: 9 in]
        n111 = case shown="True" w245 {
          tunnel: w253 -> [w310 w312]
          tunnel: [w307 w311] -> w252
          tunnel: ["CAL OFF" ("Data Out") "CAL ON" ("Data Out")] -> w254
          frame False {
            n112 = call "WSVCAP SHL Host TL RFFE Write - Multiple DUTs - Common Data.vi"("Data Out"="074044", "error in"=w310) -> ("error out"=w307:errorcluster)  [unwired: 13 in]
          }
          frame True {
            n113 = for {
              tunnel: string[] ["074900", "074920", "074900"] -> [w320] mode=indexing
              tunnel: w312 -> [w317]
              tunnel: [w316] -> w311
              n114 = call "WSVCAP SHL Host TL RFFE Write - Multiple DUTs - Common Data.vi"("Data Out"=w320, "error in"=w317, "Log (T)"=FALSE) -> ("error out"=w319:errorcluster)  [unwired: 12 in]
              n115 = call "Delay.vi"("milliseconds to wait"=u32 10, "error in (no error)"=w319) -> ("error out"=w316:errorcluster)  [unwired: 9 in]
            }
          }
        }
        n116 = for {
          N: 1 -> [_]
          tunnel: [w385] -> w284
          tunnel: w260 -> [w384]
          tunnel: w277 -> [w383]
          tunnel: "TMN DC\\CAP Data Log File Path" -> [w382]
          tunnel: w275 -> [w380]
          tunnel: [w379] -> w273
          tunnel: w270 -> [w362]
          tunnel: w269 -> [w375]
          tunnel: w266 -> [w374]
          tunnel: w263 -> [w373]
          tunnel: [w372] -> w257
          tunnel: w254 -> [w371]
          tunnel: w252 -> [w370]
          tunnel: w244 -> [w369]
          tunnel: w246 -> [w367]
          tunnel: w243 -> [w366]
          tunnel: w247 -> [w365]
          tunnel: w242 -> [w364]
          tunnel: w248 -> [w363]
          tunnel: [w362] -> w238
          tunnel: "CP Sweep" -> [w361]
          stop <- w368 stop-if-true
          n117 = while {
            tunnel: w382 -> [w596]
            tunnel: "Lot#" -> [w595]
            tunnel: "Wafer#" -> [w594]
            tunnel: w363 -> [w593]
            tunnel: "Test Program" -> [w592]
            tunnel: w363 -> [w591]
            tunnel: "Comment" -> [w590]
            tunnel: "Lot#" -> [w589]
            tunnel: "Wafer#" -> [w588]
            tunnel: w383 -> [w586]
            tunnel: [w587] -> w385
            tunnel: w384 -> [w585]
            tunnel: w380 -> [w583]
            tunnel: [w582] -> w379
            tunnel: [w503] -> w377
            tunnel: [w526] -> w376
            tunnel: w375 -> [w502]
            tunnel: w374 -> [w458]
            tunnel: w373 -> [w456]
            tunnel: [w436] -> w372
            tunnel: w371 -> [w442]
            tunnel: w370 -> [w441]
            tunnel: w369 -> [w440]
            tunnel: w367 -> [_]
            tunnel: w366 -> [w433]
            tunnel: w365 -> [w428]
            tunnel: w364 -> [w422]
            tunnel: w361 -> [w389]
            i -> [w403]
            stop <- w532 stop-if-true
            n118 = case shown="False" w389 {
              tunnel: [w600 w631] -> w455
              tunnel: [w599 w630] -> w391
              tunnel: [w598 w629] -> w454
              tunnel: w441 -> [w597 w632]
              tunnel: w403 -> [_ w628]
              frame False {
                n119 = case shown="4" "CP to HD/Cycle" {
                  selector: "CP to HD/Cycle" -> [w606 w611 w616 w621 w625]
                  tunnel: string[] ["07476F", "074776", "074765", "074769", "07477B"] -> [w607 w612 w617 w622 w627]
                  tunnel: [w605 w610 w615 w620 w626] -> w600
                  tunnel: ["35.0" ("Data Out") "27.5" ("Data Out") "30.5" ("Data Out") "44.0" ("Data Out") "40.25" ("Data Out")] -> w599
                  tunnel: [w603 w608 w613 w618 w623] -> w598
                  tunnel: w597 -> [w603 w608 w613 w618 w623]
                  frame 0, Default {
                    n120 = Index Array(array=w607, index=w606) -> (element=w605:string)
                  }
                  frame 2 {
                    n121 = Index Array(array=w612, index=w611) -> (element=w610:string)
                  }
                  frame 3 {
                    n122 = Index Array(array=w617, index=w616) -> (element=w615:string)
                  }
                  frame 4 {
                    n123 = Index Array(array=w622, index=w621) -> (element=w620:string)
                  }
                  frame 1 {
                    n124 = Index Array(array=w627, index=w625) -> (element=w626:string)
                  }
                }
              }
              frame True {
                n125 = case shown="1, Default" w628 {
                  tunnel: w632 -> [w635 w645]
                  tunnel: ["074040" w643] -> w631
                  tunnel: ["0" w642] -> w630
                  tunnel: w628 -> [_ w638]
                  tunnel: [w635 w640] -> w629
                  frame 0, 60 {
                  }
                  frame 1, Default {
                    n126 = call "WS1050 VPI CP Sweep Cmd.vi"("error in (no error)"=w645, "x"=23.0) -> ("error out"=w640:errorcluster, "Voltage Out"=w641:string[], "Cmd Out"=w644:string[])  [unwired: 5 in, 2 out]
                    n127 = Subtract(x=w638, y=1) -> (x-y=w636:i32)
                    n128 = Index Array(array=w644, index=w636) -> (element=w643:string)
                    n129 = Index Array(array=w641, index=w636) -> (element=w642:string)
                  }
                }
              }
            }
            n130 = flat-sequence {
              tunnel: [w689] -> w581
              tunnel: [w655] -> w580
              tunnel: w586 -> [w679]
              tunnel: w585 -> [w690]
              tunnel: [w690] -> w579
              tunnel: [w648] -> w578
              tunnel: [w648] -> w577
              tunnel: w454 -> [w688]
              tunnel: w403 -> [w646]
              tunnel: [w646] -> w531
              tunnel: ["Temperature"] -> w525
              tunnel: [w663] -> w520
              tunnel: [w662] -> w519
              tunnel: [w661] -> w518
              tunnel: [w666] -> w508
              tunnel: w502 -> [w687]
              tunnel: [w687] -> w501
              tunnel: [w665] -> w489
              tunnel: [w664] -> w465
              tunnel: [w686] -> w459
              tunnel: w455 -> [w657]
              tunnel: ["NA" ("Data Out")] -> w446
              tunnel: w433 -> [w674]
              tunnel: [w674] -> w432
              tunnel: w428 -> [w673]
              tunnel: [w673] -> w427
              tunnel: w422 -> [w672]
              tunnel: [w672] -> w421
              tunnel: [w669] -> w416
              tunnel: ["Test Sequences"] -> w412
              tunnel: ["WS1050/51"] -> w407
              tunnel: w391 -> [w655]
              tunnel: [w655] -> w402
              tunnel: [w657] -> w398
              tunnel: [w741] -> w500
              tunnel: w581 -> [w744]
              tunnel: w580 -> [w749]
              tunnel: [w749] -> w499
              tunnel: w579 -> [w748]
              tunnel: w578 -> [w743]
              tunnel: w577 -> [w742]
              tunnel: [w733] -> w498
              tunnel: [w748] -> w497
              tunnel: [w743] -> w496
              tunnel: [w742] -> w495
              tunnel: w531 -> [w746]
              tunnel: [w746] -> w494
              tunnel: w525 -> [w745]
              tunnel: [w745] -> w493
              tunnel: [w744] -> w492
              tunnel: w520 -> [w740]
              tunnel: w519 -> [w726]
              tunnel: w518 -> [w727]
              tunnel: w508 -> [w739]
              tunnel: [w734] -> w491
              tunnel: w501 -> [w738]
              tunnel: [w724] -> w490
              tunnel: w489 -> [w724]
              tunnel: [w726] -> w488
              tunnel: w465 -> [w725]
              tunnel: [w725] -> w464
              tunnel: [w727] -> w462
              tunnel: w459 -> [w737]
              tunnel: [w736] -> w447
              tunnel: w446 -> [w736]
              tunnel: w432 -> [w732]
              tunnel: [w732] -> w431
              tunnel: w427 -> [w731]
              tunnel: [w731] -> w426
              tunnel: w421 -> [w730]
              tunnel: [w730] -> w420
              tunnel: w416 -> [w729]
              tunnel: [w728] -> w415
              tunnel: w412 -> [w723]
              tunnel: [w723] -> w411
              tunnel: w407 -> [w722]
              tunnel: [w722] -> w406
              tunnel: w402 -> [w721]
              tunnel: [w721] -> w401
              tunnel: w398 -> [w720]
              tunnel: [w720] -> w397
              tunnel: w500 -> [w872]
              tunnel: [w871] -> w487
              tunnel: w499 -> [w882]
              tunnel: [w882] -> w484
              tunnel: w498 -> [w863]
              tunnel: [w863] -> w482
              tunnel: w497 -> [w881]
              tunnel: [w881] -> w480
              tunnel: w496 -> [w880]
              tunnel: [w880] -> w478
              tunnel: w495 -> [w879]
              tunnel: [w879] -> w476
              tunnel: w494 -> [w878]
              tunnel: [w878] -> w474
              tunnel: w493 -> [w877]
              tunnel: [w877] -> w472
              tunnel: w492 -> [w876]
              tunnel: [w876] -> w470
              tunnel: [w868] -> w468
              tunnel: w491 -> [w867]
              tunnel: w490 -> [w874]
              tunnel: w488 -> [w873]
              tunnel: w464 -> [w860]
              tunnel: [w860] -> w463
              tunnel: w462 -> [w862]
              tunnel: [w862] -> w461
              tunnel: [w869] -> w460
              tunnel: [w870] -> w448
              tunnel: w447 -> [w870]
              tunnel: w431 -> [w866]
              tunnel: [w866] -> w430
              tunnel: w426 -> [w865]
              tunnel: [w865] -> w425
              tunnel: w420 -> [w864]
              tunnel: [w864] -> w419
              tunnel: w415 -> [w861]
              tunnel: w411 -> [w859]
              tunnel: [w861] -> w410
              tunnel: [w859] -> w409
              tunnel: w406 -> [w858]
              tunnel: [w858] -> w405
              tunnel: w401 -> [w857]
              tunnel: [w857] -> w400
              tunnel: w397 -> [w856]
              tunnel: [w856] -> w396
              tunnel: w487 -> [w982]
              tunnel: [w981] -> w486
              tunnel: [w977] -> w485
              tunnel: w484 -> [w993]
              tunnel: [w993] -> w483
              tunnel: w482 -> [w971]
              tunnel: [w971] -> w481
              tunnel: w480 -> [w992]
              tunnel: [w992] -> w479
              tunnel: w478 -> [w991]
              tunnel: [w991] -> w477
              tunnel: w476 -> [w990]
              tunnel: [w990] -> w475
              tunnel: w474 -> [w989]
              tunnel: [w989] -> w473
              tunnel: w472 -> [w988]
              tunnel: [w988] -> w471
              tunnel: w470 -> [w987]
              tunnel: [w987] -> w469
              tunnel: w468 -> [w986]
              tunnel: [w986] -> w467
              tunnel: [w969] -> w466
              tunnel: w463 -> [w984]
              tunnel: w461 -> [w983]
              tunnel: w460 -> [w976]
              tunnel: ["DeltaC Target Setting(pF)"] -> w457
              tunnel: [w979] -> w449
              tunnel: w448 -> [w979]
              tunnel: w440 -> [w978]
              tunnel: [w978] -> w439
              tunnel: w430 -> [w975]
              tunnel: [w975] -> w429
              tunnel: w425 -> [w974]
              tunnel: [w974] -> w424
              tunnel: w419 -> [w973]
              tunnel: [w973] -> w418
              tunnel: w410 -> [w972]
              tunnel: w409 -> [w970]
              tunnel: [w969] -> w408
              tunnel: w405 -> [w968]
              tunnel: [w968] -> w404
              tunnel: w400 -> [w967]
              tunnel: [w967] -> w399
              tunnel: w396 -> [w966]
              tunnel: [w966] -> w395
              tunnel: [w1126] -> w576
              tunnel: [w1097] -> w575
              tunnel: w486 -> [w1130]
              tunnel: w485 -> [w1108]
              tunnel: [w1117] -> w574
              tunnel: [w1108] -> w573
              tunnel: [w1129] -> w572
              tunnel: [w1128] -> w571
              tunnel: w483 -> [w1127]
              tunnel: [w1127] -> w570
              tunnel: w481 -> [w1117]
              tunnel: w479 -> [w1125]
              tunnel: [w1125] -> w569
              tunnel: w477 -> [w1121]
              tunnel: [w1121] -> w568
              tunnel: w475 -> [w1120]
              tunnel: [w1120] -> w567
              tunnel: w473 -> [w1118]
              tunnel: [w1118] -> w530
              tunnel: w471 -> [w1124]
              tunnel: [w1124] -> w524
              tunnel: w469 -> [w1123]
              tunnel: [w1122] -> w521
              tunnel: w467 -> [w1116]
              tunnel: [w1119] -> w517
              tunnel: [w1076] -> w516
              tunnel: [w1116] -> w511
              tunnel: w466 -> [w1115]
              tunnel: [w1102] -> w507
              tunnel: [w1101] -> w506
              tunnel: [w1100] -> w505
              tunnel: w457 -> [w1114]
              tunnel: [w1099] -> w450
              tunnel: w449 -> [w1099]
              tunnel: [w1098] -> w445
              tunnel: w439 -> [_]
              tunnel: w429 -> [w1095]
              tunnel: w424 -> [w1094]
              tunnel: [w1094] -> w423
              tunnel: w418 -> [w1093]
              tunnel: [w1093] -> w417
              tunnel: w408 -> [w1090]
              tunnel: w404 -> [w1089]
              tunnel: w399 -> [w1078]
              tunnel: w395 -> [w1079]
              tunnel: [w1078] -> w394
              tunnel: w576 -> [w1285]
              tunnel: [w1285] -> w566
              tunnel: [w1270] -> w565
              tunnel: [w1284] -> w564
              tunnel: w575 -> [w1283]
              tunnel: w574 -> [w1282]
              tunnel: w573 -> [w1281]
              tunnel: [w1282] -> w563
              tunnel: [w1281] -> w562
              tunnel: w572 -> [w1280]
              tunnel: [w1280] -> w561
              tunnel: w571 -> [w1279]
              tunnel: [w1279] -> w560
              tunnel: w570 -> [w1278]
              tunnel: [w1278] -> w559
              tunnel: w569 -> [w1277]
              tunnel: [w1277] -> w558
              tunnel: w568 -> [w1276]
              tunnel: [w1276] -> w557
              tunnel: w567 -> [w1275]
              tunnel: [w1275] -> w556
              tunnel: w583 -> [w1274]
              tunnel: [w1272] -> w555
              tunnel: [w1252] -> w554
              tunnel: [w1253] -> w553
              tunnel: [w1251] -> w552
              tunnel: w530 -> [w1268]
              tunnel: [w1268] -> w529
              tunnel: w524 -> [w1267]
              tunnel: [w1267] -> w523
              tunnel: w521 -> [w1284]
              tunnel: w517 -> [w1265]
              tunnel: w516 -> [w1266]
              tunnel: [w1266] -> w515
              tunnel: [w1265] -> w513
              tunnel: w511 -> [w1264]
              tunnel: [w1264] -> w510
              tunnel: w507 -> [_]
              tunnel: w506 -> [_]
              tunnel: w505 -> [_]
              tunnel: [w1249] -> w504
              tunnel: [w1247] -> w451
              tunnel: w450 -> [w1247]
              tunnel: w445 -> [w1250]
              tunnel: [w1250] -> w444
              tunnel: w423 -> [w1249]
              tunnel: w417 -> [w1246]
              tunnel: w394 -> [w1248]
              tunnel: [w1248] -> w393
              tunnel: w566 -> [w1366]
              tunnel: [w1366] -> w551
              tunnel: w565 -> [w1387]
              tunnel: [w1386] -> w550
              tunnel: w596 -> [w1388]
              tunnel: w595 -> [w1385]
              tunnel: w594 -> [w1384]
              tunnel: w593 -> [w1383]
              tunnel: [w1382] -> w549
              tunnel: w564 -> [w1376]
              tunnel: [w1376] -> w548
              tunnel: w563 -> [w1381]
              tunnel: w562 -> [w1380]
              tunnel: [w1381] -> w547
              tunnel: [w1380] -> w546
              tunnel: [w1374] -> w545
              tunnel: w561 -> [w1379]
              tunnel: [w1379] -> w544
              tunnel: w560 -> [w1378]
              tunnel: [w1378] -> w543
              tunnel: w559 -> [w1354]
              tunnel: [w1377] -> w542
              tunnel: [w1354] -> w541
              tunnel: w558 -> [w1375]
              tunnel: w557 -> [w1373]
              tunnel: w556 -> [w1372]
              tunnel: "File Name" -> [w1371]
              tunnel: w555 -> [w1370]
              tunnel: [w1370] -> w540
              tunnel: w554 -> [w1369]
              tunnel: [w1369] -> w539
              tunnel: [w1368] -> w538
              tunnel: w553 -> [w1368]
              tunnel: w552 -> [w1367]
              tunnel: [w1367] -> w537
              tunnel: w529 -> [w1353]
              tunnel: [w1353] -> w527
              tunnel: w523 -> [w1365]
              tunnel: [w1365] -> w522
              tunnel: w515 -> [w1364]
              tunnel: [w1364] -> w514
              tunnel: w513 -> [w1363]
              tunnel: [w1363] -> w512
              tunnel: w510 -> [w1362]
              tunnel: [w1362] -> w509
              tunnel: w504 -> [w1361]
              tunnel: "NA" ("Data Out") -> [w1360]
              tunnel: [w1360] -> w453
              tunnel: [w1359] -> w452
              tunnel: w451 -> [w1359]
              tunnel: w444 -> [w1358]
              tunnel: [w1358] -> w443
              tunnel: ["Freq(Hz)"] -> w414
              tunnel: ["Board#"] -> w413
              tunnel: w393 -> [w1355]
              tunnel: [w1355] -> w392
              tunnel: w551 -> [w1455]
              tunnel: w550 -> [w1454]
              tunnel: w596 -> [w1423]
              tunnel: w592 -> [w1449]
              tunnel: w591 -> [w1452]
              tunnel: w590 -> [w1448]
              tunnel: w589 -> [w1451]
              tunnel: w588 -> [w1447]
              tunnel: w549 -> [w1450]
              tunnel: [w1455] -> w534
              tunnel: [w1453] -> w535
              tunnel: w548 -> [w1445]
              tunnel: [w1445] -> w536
              tunnel: w547 -> [w1444]
              tunnel: w546 -> [w1431]
              tunnel: w545 -> [w1443]
              tunnel: w544 -> [w1442]
              tunnel: w543 -> [w1433]
              tunnel: w542 -> [w1441]
              tunnel: w541 -> [w1440]
              tunnel: "File Name" -> [w1416]
              tunnel: w540 -> [w1439]
              tunnel: [w1439] -> w533
              tunnel: w539 -> [w1438]
              tunnel: w538 -> [w1437]
              tunnel: w537 -> [w1436]
              tunnel: [w1419] -> w528
              tunnel: w527 -> [w1419]
              tunnel: w522 -> [w1435]
              tunnel: w514 -> [w1434]
              tunnel: w512 -> [w1432]
              tunnel: w509 -> [w1430]
              tunnel: w458 -> [w1429]
              tunnel: w442 -> [w1428]
              tunnel: w456 -> [w1427]
              tunnel: w453 -> [w1426]
              tunnel: w452 -> [w1425]
              tunnel: w443 -> [w1424]
              tunnel: [w1421] -> w438
              tunnel: [w1412] -> w434
              tunnel: w414 -> [w1411]
              tunnel: w413 -> [w1409]
              tunnel: w392 -> [w1408]
              tunnel: [w1474] -> w587
              tunnel: [w1475] -> w503
              tunnel: w536 -> [w1474]
              tunnel: w535 -> [w1467]
              tunnel: w534 -> [w1475]
              tunnel: w533 -> [w1469]
              tunnel: [w1469] -> w582
              tunnel: w528 -> [w1463]
              tunnel: [w1462] -> w526
              tunnel: [w1460] -> w435
              tunnel: w438 -> [w1466]
              tunnel: w434 -> [w1464]
              frame #0 {
                n131 = call "WSVCAP SHL Host TL RFFE Write - Multiple DUTs - Common Data.vi"("Data Out"=w657, "error in"=w688, "Log (T)"=FALSE) -> ("error out"=w675:errorcluster)  [unwired: 12 in]
                n132 = for {
                  tunnel: string[] ["0760", "0767", "0768"] -> [w712] mode=indexing
                  tunnel: [w708] -> w677 mode=indexing
                  tunnel: w675 -> [w706]
                  tunnel: [w705] -> w676
                  i -> [w711]
                  n133 = call "Delay.vi"("milliseconds to wait"=u32 10, "error in (no error)"=w706) -> ("error out"=w713:errorcluster)  [unwired: 9 in]
                  n134 = call "WSVCAP SHL Host TL RFFE Read - Multiple DUTs - Common Data.vi"("Data Out"=w712, "error in"=w713, "Log (T)"=FALSE) -> ("RFFE Data In"=w710:string[], "error out"=w705:errorcluster)  [unwired: 11 in]
                  n135 = Index Array(array=w710, index=w711) -> (element=w707:string)
                  n136 = String Subset(string=w707, offset (0)=0) -> (substring=w708:string)  [unwired: 1 in]
                }
                "RB Reg for HD/Cycle" <- w677
                n137 = local read "IDD Brd(uA)"() -> (w685:string)
                n138 = call "Delay.vi"("milliseconds to wait"=u32 100, "error in (no error)"=w676) -> ("error out"=w681:errorcluster)  [unwired: 9 in]
                n139 = call "Ke2000 Single Reading.vi"("error in (no error)"=w681, "VISA resource name"=w679) -> ("error out"=w683:errorcluster, "VISA resource name out"=w660:refnum<visa-resource-name>, "uA"=w684:string)  [unwired: 5 in, 2 out]
                n140 = call "Substration.vi"("error in (no error)"=w683, "Input2"=w685, "Input1"=w684) -> ("error out"=w654:errorcluster, "In1 - In2"=→"IDD_HD/CYC (uA)":string)  [unwired: 7 in]
                n141 = case shown="0, 60" w646 {
                  tunnel: w654 -> [w695 w697 w700]
                  tunnel: [w691 w697 w703] -> w647
                  frame 0, 60 {
                    n142 = call "Delay.vi"("milliseconds to wait"=u32 10, "error in (no error)"=w695) -> ("error out"=w694:errorcluster)  [unwired: 9 in]
                    n143 = call "WSVCAP SHL Host TL RFFE Write - Multiple DUTs - Common Data.vi"("Data Out"="070201000000", "error in"=w694, "Log (T)"=FALSE) -> ("error out"=w691:errorcluster)  [unwired: 12 in]
                  }
                  frame 2, Default {
                  }
                  frame 1 {
                    n144 = call "Delay.vi"("milliseconds to wait"=u32 10, "error in (no error)"=w700) -> ("error out"=w699:errorcluster)  [unwired: 9 in]
                    n145 = call "WSVCAP SHL Host TL RFFE Write - Multiple DUTs - Common Data.vi"("Data Out"="0702013B3B3B", "error in"=w699, "Log (T)"=FALSE) -> ("error out"=w703:errorcluster)  [unwired: 12 in]
                  }
                }
                n146 = flat-sequence {
                  tunnel: w671 -> [w715]
                  tunnel: [w715] -> w668
                  frame #0 {
                    w716 = "0" ("NOM IDD OFF(uA)")
                    w717 = string[] []
                    w718 = string[][] []
                    n147 = local write "NOM IDD ON (uA)"(w716) -> ()
                    n148 = local write "Total Delta C1(pF)"(w717) -> ()
                    n149 = local write "Total Delta C2(pF)"(w717) -> ()
                    n150 = local write "Total Delta C3(pF)"(w717) -> ()
                    n151 = local write "Current EFuse Read back"(w717) -> ()
                    n152 = local write "RB Reg for HD/Cycle"(w717) -> ()
                    n153 = local write "NOM IDD OFF(uA)"(w716) -> ()
                    n154 = local write "VSA_V3"(w718) -> ()
                    n155 = local write "VSA_V1"(w718) -> ()
                    n156 = local write "VSA_V2"(w718) -> ()
                    n157 = local write "VPI C1"(w718) -> ()
                    n158 = local write "VPI C2"(w718) -> ()
                    n159 = local write "VPI C3"(w718) -> ()
                    n160 = local write "% Delta C"(w718) -> ()
                    n161 = local write "40V_3"(w718) -> ()
                    n162 = local write "40V_2"(w718) -> ()
                    n163 = local write "40V_1"(w718) -> ()
                  }
                }
                n164 = local read "IDD Brd(uA)"() -> (w649:string)
                n165 = call "Delay.vi"("milliseconds to wait"=u32 100, "error in (no error)"=w647) -> ("error out"=w652:errorcluster)  [unwired: 9 in]
                n166 = call "Ke2000 Single Reading.vi"("error in (no error)"=w652, "VISA resource name"=w660) -> ("error out"=w651:errorcluster, "VISA resource name out"=w689:refnum<visa-resource-name>, "uA"=w650:string)  [unwired: 5 in, 2 out]
                n167 = call "Substration.vi"("error in (no error)"=w651, "Input2"=w649, "Input1"=w650) -> ("error out"=w671:errorcluster, "In1 - In2"=w648:string)  [unwired: 7 in]
                n168 = local read "Clock Rate (Hz)"() -> (w686:dbl)
                n169 = call "Multi Dut Cmd_Header Setting.vi"("WS1050/51"="WS1050/51", "Test Seq"="Test Sequences", "error in (no error)"=w668) -> ("Name 1"=w666:string[], "Name 2"=w665:string[], "Name 3"=w664:string[], "Cmd 3"=w661:string[], "Cmd 1"=w663:string[], "Cmd 2"=w662:string[], "error out"=w669:errorcluster)  [unwired: 3 in, 3 out]
              }
              frame #1 {
                w728 = FALSE ("Log (T)")
                n170 = call "WSVCAP SHL Host TL RFFE Configure.vi"("RFFE Slave Address"=w738, "Clock Rate (Hz)"=w737, "error in"=w729) -> ("Actual Rate (Hz)"=w747:dbl, "error out"=w735:errorcluster)  [unwired: 11 in]
                n171 = local write "AR  Measurent(Hz)"(w747) -> ()
                n172 = Array Size(array=w739) -> (size(s)=w750:i32)
                n173 = case shown="True" FALSE {
                  tunnel: w750 -> [_ w763]
                  tunnel: [_ w762] -> w741
                  tunnel: w740 -> [_ w761]
                  tunnel: w739 -> [_ w760]
                  tunnel: w735 -> [w752 w759]
                  tunnel: [w752 w758] -> w734
                  tunnel: [string[][] [] w757] -> w733
                  tunnel: w728 -> [_ w756]
                  tunnel: w723 -> [_ w754]
                  tunnel: w721 -> [_ w753]
                  frame False {
                  }
                  frame True {
                    n174 = case shown="0, Default" w754 {
                      tunnel: w763 -> [w772 w804 w833]
                      tunnel: [w771 w803 w832] -> w762
                      tunnel: w761 -> [w770 w802 w831]
                      tunnel: w760 -> [w769 w801 w830]
                      tunnel: w759 -> [w768 w800 w829]
                      tunnel: [w767 w799 w828] -> w758
                      tunnel: w756 -> [w766 w798 w827]
                      tunnel: [w765 w797 w826] -> w755
                      tunnel: w753 -> [w764 _ _]
                      frame 0, Default {
                        n175 = for {
                          N: w772 -> [_]
                          tunnel: w770 -> [w792]
                          tunnel: [w773] -> w771
                          tunnel: [w789] -> w765 mode=indexing
                          tunnel: w769 -> [w790]
                          tunnel: w768 -> [w779]
                          tunnel: [w781] -> w767
                          tunnel: w766 -> [w780]
                          tunnel: w764 -> [w774]
                          i -> [w788]
                          stop <- w773 stop-if-true
                          n176 = Index Array(array=w792, index=w788) -> (element=w791:string)
                          n177 = Index Array(array=w790, index=w788) -> (element=w776:string)
                          n178 = call <vilib>:"Space Constant.vi"() -> ("String"=w775:string)
                          n179 = call "WSVCAP SHL Host TL RFFE Write - Multiple DUTs - Common Data.vi"("Data Out"=w791, "error in"=w779, "Log (T)"=FALSE) -> ("error out"=w783:errorcluster)  [unwired: 12 in]
                          n180 = Concatenate Strings(w776, w775, w774) -> (w777:string)
                          n181 = call "Delay.vi"("milliseconds to wait"=u32 10, "error in (no error)"=w783) -> ("error out"=w787:errorcluster)  [unwired: 9 in]
                          n182 = call "WS1050 AD7747 READ 36 DUT.vi"("error in"=w787, "Log (T)"=w780, "DUT Mask Mode (All)"=WSVCAP_SHL_I2C_DUT_Mask_Mode_Enum."C1") -> ("error out"=w785:errorcluster, "AD7747 Values"=w786:string[][])  [unwired: 7 in]
                          n183 = local write "STATUS"(w777) -> ()
                          n184 = for {
                            tunnel: w786 -> [w795] mode=indexing
                            tunnel: w785 -> [w796]
                            tunnel: [w796] -> w781
                            tunnel: [w793] -> w789 mode=indexing
                            n185 = Index Array(array=w795, index=1) -> (element=w793:string)
                          }
                          n186 = Unbundle By Name(w781) -> ("status"=w773:bool)
                        }
                      }
                      frame 1 {
                        n187 = for {
                          N: w804 -> [_]
                          tunnel: w802 -> [w821]
                          tunnel: [w805] -> w803
                          tunnel: [w817] -> w797 mode=indexing
                          tunnel: w801 -> [w819]
                          tunnel: w800 -> [w807]
                          tunnel: [w809] -> w799
                          tunnel: w798 -> [w808]
                          i -> [w816]
                          stop <- w805 stop-if-true
                          n188 = Index Array(array=w821, index=w816) -> (element=w820:string)
                          n189 = Index Array(array=w819, index=w816) -> (element=w818:string)
                          n190 = local write "STATUS"(w818) -> ()
                          n191 = call "WSVCAP SHL Host TL RFFE Write - Multiple DUTs - Common Data.vi"("Data Out"=w820, "error in"=w807, "Log (T)"=FALSE) -> ("error out"=w811:errorcluster)  [unwired: 12 in]
                          n192 = call "Delay.vi"("milliseconds to wait"=u32 10, "error in (no error)"=w811) -> ("error out"=w815:errorcluster)  [unwired: 9 in]
                          n193 = call "WS1050 AD7747 READ 36 DUT.vi"("error in"=w815, "Log (T)"=w808, "DUT Mask Mode (All)"=WSVCAP_SHL_I2C_DUT_Mask_Mode_Enum."C2") -> ("error out"=w813:errorcluster, "AD7747 Values"=w814:string[][])  [unwired: 7 in]
                          n194 = for {
                            tunnel: w814 -> [w824] mode=indexing
                            tunnel: w813 -> [w825]
                            tunnel: [w825] -> w809
                            tunnel: [w822] -> w817 mode=indexing
                            n195 = Index Array(array=w824, index=3) -> (element=w822:string)
                          }
                          n196 = Unbundle By Name(w809) -> ("status"=w805:bool)
                        }
                      }
                      frame 2 {
                        n197 = for {
                          N: w833 -> [_]
                          tunnel: w831 -> [w850]
                          tunnel: [w834] -> w832
                          tunnel: [w846] -> w826 mode=indexing
                          tunnel: w830 -> [w848]
                          tunnel: w829 -> [w836]
                          tunnel: [w838] -> w828
                          tunnel: w827 -> [w837]
                          i -> [w845]
                          stop <- w834 stop-if-true
                          n198 = Index Array(array=w850, index=w845) -> (element=w849:string)
                          n199 = Index Array(array=w848, index=w845) -> (element=w847:string)
                          n200 = local write "STATUS"(w847) -> ()
                          n201 = call "WSVCAP SHL Host TL RFFE Write - Multiple DUTs - Common Data.vi"("Data Out"=w849, "error in"=w836, "Log (T)"=FALSE) -> ("error out"=w840:errorcluster)  [unwired: 12 in]
                          n202 = call "Delay.vi"("milliseconds to wait"=u32 10, "error in (no error)"=w840) -> ("error out"=w844:errorcluster)  [unwired: 9 in]
                          n203 = call "WS1050 AD7747 READ 36 DUT.vi"("error in"=w844, "Log (T)"=w837, "DUT Mask Mode (All)"=WSVCAP_SHL_I2C_DUT_Mask_Mode_Enum."C3") -> ("error out"=w842:errorcluster, "AD7747 Values"=w843:string[][])  [unwired: 7 in]
                          n204 = for {
                            tunnel: w843 -> [w853] mode=indexing
                            tunnel: w842 -> [w854]
                            tunnel: [w854] -> w838
                            tunnel: [w851] -> w846 mode=indexing
                            n205 = Index Array(array=w853, index=5) -> (element=w851:string)
                          }
                          n206 = Unbundle By Name(w838) -> ("status"=w834:bool)
                        }
                      }
                    }
                    n207 = Transpose 2D Array(2D array=w755) -> (transposed array=w757:string[][])
                    "40V_1" <- w757
                  }
                }
                "NOM IDD ON (uA)" <- w743
                "NOM IDD OFF(uA)" <- w742
              }
              frame #2 {
                n208 = Array Size(array=w874) -> (size(s)=w875:i32)
                n209 = case shown="False" FALSE {
                  tunnel: w875 -> [_ w896]
                  tunnel: w874 -> [_ w895]
                  tunnel: w873 -> [_ w894]
                  tunnel: w872 -> [_ w893]
                  tunnel: [_ w892] -> w871
                  tunnel: [w884 w891] -> w869
                  tunnel: [string[][] [] w890] -> w868
                  tunnel: w867 -> [w884 w889]
                  tunnel: w861 -> [_ w888]
                  tunnel: w859 -> [_ w886]
                  tunnel: w857 -> [_ w885]
                  frame False {
                  }
                  frame True {
                    n210 = case shown="0, 2, Default" w886 {
                      tunnel: w896 -> [w906 w941]
                      tunnel: w895 -> [w905 w940]
                      tunnel: w894 -> [w904 w939]
                      tunnel: w893 -> [w903 w938]
                      tunnel: [w902 w937] -> w892
                      tunnel: [w901 w936] -> w891
                      tunnel: w889 -> [w900 w935]
                      tunnel: w888 -> [w899 w934]
                      tunnel: [w898 w933] -> w887
                      tunnel: w885 -> [w897 _]
                      frame 0, 2, Default {
                        n211 = for {
                          N: w906 -> [_]
                          tunnel: w904 -> [w928]
                          tunnel: w903 -> [w926]
                          tunnel: [w925] -> w902
                          tunnel: [w922] -> w898 mode=indexing
                          tunnel: w905 -> [w923]
                          tunnel: w900 -> [w912]
                          tunnel: [w914] -> w901
                          tunnel: w899 -> [w913]
                          tunnel: w897 -> [w907]
                          i -> [w921]
                          stop <- w925 stop-if-true
                          n212 = Index Array(array=w928, index=w921) -> (element=w924:string)
                          n213 = Index Array(array=w923, index=w921) -> (element=w908:string)
                          n214 = call <vilib>:"Space Constant.vi"() -> ("String"=w909:string)
                          n215 = call "WSVCAP SHL Host TL RFFE Write - Multiple DUTs - Common Data.vi"("Data Out"=w924, "error in"=w912, "Log (T)"=FALSE) -> ("error out"=w916:errorcluster)  [unwired: 12 in]
                          n216 = Concatenate Strings(w908, w909, w907) -> (w910:string)
                          n217 = call "Delay.vi"("milliseconds to wait"=u32 10, "error in (no error)"=w916) -> ("error out"=w920:errorcluster)  [unwired: 9 in]
                          n218 = call "WS1050 AD7747 READ 36 DUT.vi"("error in"=w920, "Log (T)"=w913, "DUT Mask Mode (All)"=WSVCAP_SHL_I2C_DUT_Mask_Mode_Enum."C2") -> ("error out"=w918:errorcluster, "AD7747 Values"=w919:string[][])  [unwired: 7 in]
                          n219 = local write "STATUS"(w910) -> ()
                          n220 = for {
                            tunnel: w919 -> [w931] mode=indexing
                            tunnel: w918 -> [w932]
                            tunnel: [w932] -> w914
                            tunnel: [w929] -> w922 mode=indexing
                            n221 = Index Array(array=w931, index=3) -> (element=w929:string)
                          }
                          n222 = Unbundle By Name(w914) -> ("status"=w927:bool)
                          n223 = Or(x=w927, y=w926) -> (x .or. y?=w925:bool)
                        }
                      }
                      frame 1 {
                        n224 = for {
                          N: w941 -> [_]
                          tunnel: w939 -> [w960]
                          tunnel: w938 -> [w958]
                          tunnel: [w957] -> w937
                          tunnel: [w953] -> w933 mode=indexing
                          tunnel: w940 -> [w955]
                          tunnel: w935 -> [w943]
                          tunnel: [w945] -> w936
                          tunnel: w934 -> [w944]
                          i -> [w952]
                          stop <- w957 stop-if-true
                          n225 = Index Array(array=w960, index=w952) -> (element=w956:string)
                          n226 = Index Array(array=w955, index=w952) -> (element=w954:string)
                          n227 = call "WSVCAP SHL Host TL RFFE Write - Multiple DUTs - Common Data.vi"("Data Out"=w956, "error in"=w943, "Log (T)"=FALSE) -> ("error out"=w947:errorcluster)  [unwired: 12 in]
                          n228 = local write "STATUS"(w954) -> ()
                          n229 = call "Delay.vi"("milliseconds to wait"=u32 10, "error in (no error)"=w947) -> ("error out"=w951:errorcluster)  [unwired: 9 in]
                          n230 = call "WS1050 AD7747 READ 36 DUT.vi"("error in"=w951, "Log (T)"=w944, "DUT Mask Mode (All)"=WSVCAP_SHL_I2C_DUT_Mask_Mode_Enum."C1") -> ("error out"=w949:errorcluster, "AD7747 Values"=w950:string[][])  [unwired: 7 in]
                          n231 = for {
                            tunnel: w950 -> [w963] mode=indexing
                            tunnel: w949 -> [w964]
                            tunnel: [w964] -> w945
                            tunnel: [w961] -> w953 mode=indexing
                            n232 = Index Array(array=w963, index=1) -> (element=w961:string)
                          }
                          n233 = Unbundle By Name(w945) -> ("status"=w959:bool)
                          n234 = Or(x=w959, y=w958) -> (x .or. y?=w957:bool)
                        }
                      }
                    }
                    n235 = Transpose 2D Array(2D array=w887) -> (transposed array=w890:string[][])
                    "40V_2" <- w890
                  }
                }
              }
              frame #3 {
                n236 = Array Size(array=w984) -> (size(s)=w985:i32)
                n237 = case shown="False" FALSE {
                  tunnel: w985 -> [_ w1007]
                  tunnel: w984 -> [_ w1006]
                  tunnel: w983 -> [_ w1005]
                  tunnel: w982 -> [_ w1004]
                  tunnel: [_ w1003] -> w981
                  tunnel: [string[][] [] w1002] -> w977
                  tunnel: w976 -> [w995 w1001]
                  tunnel: w972 -> [_ w1000]
                  tunnel: w970 -> [_ w998]
                  tunnel: [w995 w997] -> w969
                  tunnel: w967 -> [_ w996]
                  frame False {
                  }
                  frame True {
                    n238 = case shown="2" w998 {
                      tunnel: w1007 -> [w1017 w1052]
                      tunnel: w1006 -> [w1016 w1051]
                      tunnel: w1005 -> [w1015 w1050]
                      tunnel: w1004 -> [w1014 w1049]
                      tunnel: [w1013 w1048] -> w1003
                      tunnel: w1001 -> [w1012 w1047]
                      tunnel: [w1011 w1046] -> w997
                      tunnel: w1000 -> [w1010 w1045]
                      tunnel: [w1009 w1044] -> w999
                      tunnel: w996 -> [w1008 _]
                      frame 0, 1, Default {
                        n239 = for {
                          N: w1017 -> [_]
                          tunnel: w1015 -> [w1039]
                          tunnel: w1014 -> [w1037]
                          tunnel: [w1036] -> w1013
                          tunnel: [w1033] -> w1009 mode=indexing
                          tunnel: w1016 -> [w1034]
                          tunnel: w1012 -> [w1023]
                          tunnel: [w1025] -> w1011
                          tunnel: w1010 -> [w1024]
                          tunnel: w1008 -> [w1018]
                          i -> [w1032]
                          stop <- w1036 stop-if-true
                          n240 = Index Array(array=w1039, index=w1032) -> (element=w1035:string)
                          n241 = Index Array(array=w1034, index=w1032) -> (element=w1020:string)
                          n242 = call <vilib>:"Space Constant.vi"() -> ("String"=w1019:string)
                          n243 = call "WSVCAP SHL Host TL RFFE Write - Multiple DUTs - Common Data.vi"("Data Out"=w1035, "error in"=w1023, "Log (T)"=FALSE) -> ("error out"=w1027:errorcluster)  [unwired: 12 in]
                          n244 = call "Delay.vi"("milliseconds to wait"=u32 10, "error in (no error)"=w1027) -> ("error out"=w1031:errorcluster)  [unwired: 9 in]
                          n245 = Concatenate Strings(w1020, w1019, w1018) -> (w1021:string)
                          n246 = call "WS1050 AD7747 READ 36 DUT.vi"("error in"=w1031, "Log (T)"=w1024, "DUT Mask Mode (All)"=WSVCAP_SHL_I2C_DUT_Mask_Mode_Enum."C3") -> ("error out"=w1029:errorcluster, "AD7747 Values"=w1030:string[][])  [unwired: 7 in]
                          n247 = for {
                            tunnel: w1030 -> [w1042] mode=indexing
                            tunnel: w1029 -> [w1043]
                            tunnel: [w1043] -> w1025
                            tunnel: [w1040] -> w1033 mode=indexing
                            n248 = Index Array(array=w1042, index=5) -> (element=w1040:string)
                          }
                          n249 = Unbundle By Name(w1025) -> ("status"=w1038:bool)
                          n250 = local write "STATUS"(w1021) -> ()
                          n251 = Or(x=w1038, y=w1037) -> (x .or. y?=w1036:bool)
                        }
                      }
                      frame 2 {
                        n252 = for {
                          N: w1052 -> [_]
                          tunnel: w1050 -> [w1071]
                          tunnel: w1049 -> [w1069]
                          tunnel: [w1068] -> w1048
                          tunnel: [w1064] -> w1044 mode=indexing
                          tunnel: w1051 -> [w1066]
                          tunnel: w1047 -> [w1054]
                          tunnel: [w1056] -> w1046
                          tunnel: w1045 -> [w1055]
                          i -> [w1063]
                          stop <- w1068 stop-if-true
                          n253 = Index Array(array=w1071, index=w1063) -> (element=w1067:string)
                          n254 = Index Array(array=w1066, index=w1063) -> (element=w1065:string)
                          n255 = local write "STATUS"(w1065) -> ()
                          n256 = call "WSVCAP SHL Host TL RFFE Write - Multiple DUTs - Common Data.vi"("Data Out"=w1067, "error in"=w1054, "Log (T)"=FALSE) -> ("error out"=w1058:errorcluster)  [unwired: 12 in]
                          n257 = call "Delay.vi"("milliseconds to wait"=u32 10, "error in (no error)"=w1058) -> ("error out"=w1062:errorcluster)  [unwired: 9 in]
                          n258 = call "WS1050 AD7747 READ 36 DUT.vi"("error in"=w1062, "Log (T)"=w1055, "DUT Mask Mode (All)"=WSVCAP_SHL_I2C_DUT_Mask_Mode_Enum."C1") -> ("error out"=w1060:errorcluster, "AD7747 Values"=w1061:string[][])  [unwired: 7 in]
                          n259 = for {
                            tunnel: w1061 -> [w1074] mode=indexing
                            tunnel: w1060 -> [w1075]
                            tunnel: [w1075] -> w1056
                            tunnel: [w1072] -> w1064 mode=indexing
                            n260 = Index Array(array=w1074, index=1) -> (element=w1072:string)
                          }
                          n261 = Unbundle By Name(w1056) -> ("status"=w1070:bool)
                          n262 = Or(x=w1070, y=w1069) -> (x .or. y?=w1068:bool)
                        }
                      }
                    }
                    n263 = Transpose 2D Array(2D array=w999) -> (transposed array=w1002:string[][])
                    "40V_3" <- w1002
                  }
                }
              }
              frame #4 {
                # "VPI Testing @ 35V"
                n264 = call "WS1050 Delta C Calculation.vi"("error in (no error)"=w1115, "DCap Target(pF)"=w1114, "Input"=w1117) -> ("error out"=w1112:errorcluster, "Total Bank Delta C(pF)"=w1105:string[], "% Bank DeltaC"=w1109:string[])  [unwired: 3 in, 3 out]
                n265 = call "WS1050 Delta C Calculation.vi"("error in (no error)"=w1115, "DCap Target(pF)"=w1114, "Input"=w1116) -> ("error out"=w1113:errorcluster, "Total Bank Delta C(pF)"=w1104:string[], "% Bank DeltaC"=w1107:string[])  [unwired: 3 in, 3 out]
                n266 = call "WS1050 Delta C Calculation.vi"("error in (no error)"=w1115, "DCap Target(pF)"=w1114, "Input"=w1108) -> ("error out"=w1111:errorcluster, "Total Bank Delta C(pF)"=w1103:string[], "% Bank DeltaC"=w1106:string[])  [unwired: 3 in, 3 out]
                n267 = call "WS1050_51 VPI Header CV Curve.vi"("error in (no error)"=w1090, "WS1050/51"=w1089, "VPI_Cmd"="VPI_Cmd", "VPI Name"="VPI Name") -> ("error out"=w1082:errorcluster, "Cmd_3"=w1083:string[], "VPI_3"=w1086:string[], "VPI Header"=w1076:string[], "Cmd_2"=w1084:string[], "VPI_2"=w1087:string[], "Cmd_1"=w1085:string[], "VPI_1"=w1088:string[])
                n268 = Merge Errors(w1112, w1113, w1111) -> (w1110:errorcluster)
                n269 = case shown="1, Default" w1118 {
                  tunnel: w1110 -> [w1138 w1146]
                  tunnel: [w1138 w1146] -> w1081
                  tunnel: w1109 -> [w1134 w1142]
                  tunnel: w1107 -> [w1133 w1141]
                  tunnel: w1106 -> [w1132 w1140]
                  tunnel: w1105 -> [w1137 w1145]
                  tunnel: [w1137 w1145] -> w1102
                  tunnel: w1104 -> [w1136 w1144]
                  tunnel: [w1136 w1144] -> w1101
                  tunnel: w1103 -> [w1135 w1143]
                  tunnel: [w1135 w1143] -> w1100
                  frame 0 {
                    n270 = Build Array(w1134, w1133, w1132) -> (→"% Delta C_T0":string[][])
                  }
                  frame 1, Default {
                    n271 = Build Array(w1142, w1141, w1140) -> (→"% Delta C":string[][])
                  }
                }
                "Total Delta C1(pF)" <- w1102
                "Total Delta C2(pF)" <- w1101
                "Total Delta C3(pF)" <- w1100
                n272 = Merge Errors(w1082, w1081) -> (w1080:errorcluster)
                n273 = case shown="True" w1095 {
                  tunnel: w1130 -> [w1149 w1175]
                  tunnel: [w1148 w1167] -> w1077
                  tunnel: [w1147 w1156] -> w1129
                  tunnel: [w1147 w1154] -> w1128
                  tunnel: [w1149 w1168] -> w1126
                  tunnel: w1123 -> [w1151 w1176]
                  tunnel: [w1151 w1176] -> w1122
                  tunnel: w1085 -> [_ w1174]
                  tunnel: w1084 -> [_ w1171]
                  tunnel: w1083 -> [_ w1169]
                  tunnel: [w1147 w1155] -> w1119
                  tunnel: w1088 -> [_ w1173]
                  tunnel: w1087 -> [_ w1172]
                  tunnel: w1086 -> [_ w1170]
                  tunnel: ["NA" ("string") w1153] -> w1098
                  tunnel: w1080 -> [w1148 w1152]
                  tunnel: w1078 -> [_ w1153]
                  tunnel: w1079 -> [_ _]
                  frame False {
                    w1147 = string[][] []
                  }
                  frame True {
                    n274 = Array Size(array=w1173) -> (size(s)=w1157:i32)
                    n275 = for {
                      N: w1157 -> [_]
                      tunnel: w1174 -> [w1241]
                      tunnel: w1175 -> [w1239]
                      tunnel: [w1238] -> w1164
                      tunnel: [w1237] -> w1166 mode=indexing
                      tunnel: w1173 -> [w1236]
                      tunnel: w1152 -> [w1223]
                      tunnel: [w1229] -> w1159
                      tunnel: w1153 -> [w1224]
                      i -> [w1235]
                      stop <- w1238 stop-if-true
                      (unwired) FALSE ("Log (T)")
                      n276 = Index Array(array=w1241, index=w1235) -> ()  [unwired: 1 out]
                      n277 = Index Array(array=w1236, index=w1235) -> (element=w1227:string)
                      n278 = call <vilib>:"Space Constant.vi"() -> ("String"=w1225:string)
                      n279 = Concatenate Strings(w1227, w1225, w1224) -> (w1226:string)
                      n280 = call "Delay.vi"("milliseconds to wait"=u32 10, "error in (no error)"=w1223) -> ("error out"=w1231:errorcluster)  [unwired: 9 in]
                      n281 = local write "STATUS"(w1226) -> ()
                      n282 = call "WS1050 AD7747 READ 36 DUT.vi"("error in"=w1231, "Log (T)"=FALSE, "DUT Mask Mode (All)"=WSVCAP_SHL_I2C_DUT_Mask_Mode_Enum."C1") -> ("error out"=w1233:errorcluster, "AD7747 Values"=w1232:string[][])  [unwired: 7 in]
                      n283 = for {
                        tunnel: [w1244] -> w1237 mode=indexing
                        tunnel: w1233 -> [w1243]
                        tunnel: [w1243] -> w1229
                        tunnel: w1232 -> [w1242] mode=indexing
                        n284 = Index Array(array=w1242, index=1) -> (element=w1244:string)
                      }
                      n285 = Unbundle By Name(w1229) -> ("status"=w1240:bool)
                      n286 = Or(x=w1240, y=w1239) -> (x .or. y?=w1238:bool)
                    }
                    n287 = Transpose 2D Array(2D array=w1166) -> (transposed array=w1156:string[][])
                    "VPI C1" <- w1156
                    n288 = Array Size(array=w1172) -> (size(s)=w1165:i32)
                    n289 = for {
                      N: w1165 -> [_]
                      tunnel: w1171 -> [w1218]
                      tunnel: w1164 -> [w1216]
                      tunnel: [w1215] -> w1160
                      tunnel: [w1214] -> w1163 mode=indexing
                      tunnel: w1172 -> [w1213]
                      tunnel: w1159 -> [w1200]
                      tunnel: [w1206] -> w1158
                      tunnel: w1153 -> [w1202]
                      i -> [w1212]
                      stop <- w1215 stop-if-true
                      (unwired) FALSE ("Log (T)")
                      n290 = Index Array(array=w1218, index=w1212) -> ()  [unwired: 1 out]
                      n291 = Index Array(array=w1213, index=w1212) -> (element=w1204:string)
                      n292 = call <vilib>:"Space Constant.vi"() -> ("String"=w1203:string)
                      n293 = Concatenate Strings(w1204, w1203, w1202) -> (w1201:string)
                      n294 = call "Delay.vi"("milliseconds to wait"=u32 10, "error in (no error)"=w1200) -> ("error out"=w1208:errorcluster)  [unwired: 9 in]
                      n295 = call "WS1050 AD7747 READ 36 DUT.vi"("error in"=w1208, "Log (T)"=FALSE, "DUT Mask Mode (All)"=WSVCAP_SHL_I2C_DUT_Mask_Mode_Enum."C2") -> ("error out"=w1210:errorcluster, "AD7747 Values"=w1209:string[][])  [unwired: 7 in]
                      n296 = local write "STATUS"(w1201) -> ()
                      n297 = for {
                        tunnel: [w1221] -> w1214 mode=indexing
                        tunnel: w1210 -> [w1220]
                        tunnel: [w1220] -> w1206
                        tunnel: w1209 -> [w1219] mode=indexing
                        n298 = Index Array(array=w1219, index=3) -> (element=w1221:string)
                      }
                      n299 = Unbundle By Name(w1206) -> ("status"=w1217:bool)
                      n300 = Or(x=w1217, y=w1216) -> (x .or. y?=w1215:bool)
                    }
                    n301 = Transpose 2D Array(2D array=w1163) -> (transposed array=w1155:string[][])
                    "VPI C2" <- w1155
                    n302 = Array Size(array=w1170) -> (size(s)=w1162:i32)
                    n303 = for {
                      N: w1162 -> [_]
                      tunnel: w1169 -> [w1195]
                      tunnel: w1160 -> [w1193]
                      tunnel: [w1192] -> w1168
                      tunnel: [w1191] -> w1161 mode=indexing
                      tunnel: w1170 -> [w1190]
                      tunnel: w1158 -> [w1177]
                      tunnel: [w1183] -> w1167
                      tunnel: w1153 -> [w1179]
                      i -> [w1189]
                      stop <- w1192 stop-if-true
                      (unwired) FALSE ("Log (T)")
                      n304 = Index Array(array=w1195, index=w1189) -> ()  [unwired: 1 out]
                      n305 = Index Array(array=w1190, index=w1189) -> (element=w1181:string)
                      n306 = call <vilib>:"Space Constant.vi"() -> ("String"=w1178:string)
                      n307 = call "Delay.vi"("milliseconds to wait"=u32 10, "error in (no error)"=w1177) -> ("error out"=w1185:errorcluster)  [unwired: 9 in]
                      n308 = Concatenate Strings(w1181, w1178, w1179) -> (w1180:string)
                      n309 = call "WS1050 AD7747 READ 36 DUT.vi"("error in"=w1185, "Log (T)"=FALSE, "DUT Mask Mode (All)"=WSVCAP_SHL_I2C_DUT_Mask_Mode_Enum."C3") -> ("error out"=w1187:errorcluster, "AD7747 Values"=w1186:string[][])  [unwired: 7 in]
                      n310 = local write "STATUS"(w1180) -> ()
                      n311 = for {
                        tunnel: [w1198] -> w1191 mode=indexing
                        tunnel: w1187 -> [w1197]
                        tunnel: [w1197] -> w1183
                        tunnel: w1186 -> [w1196] mode=indexing
                        n312 = Index Array(array=w1196, index=5) -> (element=w1198:string)
                      }
                      n313 = Unbundle By Name(w1183) -> ("status"=w1194:bool)
                      n314 = Or(x=w1194, y=w1193) -> (x .or. y?=w1192:bool)
                    }
                    n315 = Transpose 2D Array(2D array=w1161) -> (transposed array=w1154:string[][])
                    "VPI C3" <- w1154
                  }
                }
                n316 = call "Delay.vi"("milliseconds to wait"=u32 10, "error in (no error)"=w1077) -> ("error out"=w1097:errorcluster)  [unwired: 9 in]
              }
              frame #5 {
                n317 = case shown="True" w1246 {
                  tunnel: w1283 -> [w1297 w1299]
                  tunnel: [w1297 w1298] -> w1257
                  tunnel: [w1296 w1305] -> w1273
                  tunnel: w1274 -> [w1296 w1304]
                  tunnel: [w1294 w1302] -> w1262
                  tunnel: [w1294 w1301] -> w1259
                  tunnel: [w1294 w1300] -> w1256
                  tunnel: [string[][] [] w1303] -> w1263
                  frame False {
                    w1294 = string[][] []
                  }
                  frame True {
                    n318 = for {
                      tunnel: "VSA Voltage(V)" -> [w1329] mode=indexing
                      tunnel: [w1333] -> w1305
                      tunnel: w1304 -> [w1331]
                      tunnel: [w1330] -> w1302 mode=indexing
                      tunnel: [w1317] -> w1301 mode=indexing
                      tunnel: [w1326] -> w1303 mode=indexing
                      tunnel: [w1311] -> w1300 mode=indexing
                      tunnel: w1299 -> [w1310]
                      tunnel: [w1309] -> w1298
                      w1308 = FALSE ("Log (T)")
                      w1325 = u16 0 items=["Voltage", "Current"] ("Source Mode  (0: Voltage)")
                      n319 = call "Ke2400 Configure Output.vi"("Source Mode  (0: Voltage)"=w1325, "error in (no error)"=w1310, "Compliance  Level (0.1)"=0.1, "Output Level (0)"=w1329, "VISA resource name"=w1331) -> ("error out"=w1337:errorcluster, "VISA resource name out"=w1335:refnum<visa-resource-name>)  [unwired: 5 in]
                      n320 = Number To Fractional String(number=w1329) -> (F-format string=w1328:string)  [unwired: 3 in]
                      n321 = call "Ke2400 Enable.vi"("error in (no error)"=w1337, "ON/OFF"=TRUE ("Enable Output (T: Enable)"), "VISA resource name"=w1335) -> ("error out"=w1338:errorcluster, "VISA resource name out"=w1333:refnum<visa-resource-name>)  [unwired: 7 in]
                      n322 = call "Delay.vi"("milliseconds to wait"=u32 10, "error in (no error)"=w1338) -> ("error out"=w1324:errorcluster)  [unwired: 9 in]
                      n323 = call "WS1050 AD7747 READ 36 DUT.vi"("error in"=w1324, "Log (T)"=w1308, "DUT Mask Mode (All)"=WSVCAP_SHL_I2C_DUT_Mask_Mode_Enum."C1") -> ("error out"=w1321:errorcluster, "AD7747 Values"=w1323:string[][])  [unwired: 7 in]
                      n324 = for {
                        tunnel: w1323 -> [w1349] mode=indexing
                        tunnel: [w1350] -> w1330 mode=indexing
                        tunnel: w1321 -> [w1348]
                        tunnel: [w1348] -> w1320
                        n325 = Index Array(array=w1349, index=1) -> (element=w1350:string)
                      }
                      n326 = for {
                        N: 36 -> [_]
                        tunnel: w1328 -> [w1347]
                        tunnel: [w1347] -> w1326 mode=indexing
                      }
                      n327 = call "WS1050 AD7747 READ 36 DUT.vi"("error in"=w1320, "Log (T)"=w1308, "DUT Mask Mode (All)"=WSVCAP_SHL_I2C_DUT_Mask_Mode_Enum."C2") -> ("error out"=w1318:errorcluster, "AD7747 Values"=w1316:string[][])  [unwired: 7 in]
                      n328 = for {
                        tunnel: w1316 -> [w1344] mode=indexing
                        tunnel: [w1345] -> w1317 mode=indexing
                        tunnel: w1318 -> [w1343]
                        tunnel: [w1343] -> w1315
                        n329 = Index Array(array=w1344, index=3) -> (element=w1345:string)
                      }
                      n330 = call "WS1050 AD7747 READ 36 DUT.vi"("error in"=w1315, "Log (T)"=w1308, "DUT Mask Mode (All)"=WSVCAP_SHL_I2C_DUT_Mask_Mode_Enum."C3") -> ("error out"=w1313:errorcluster, "AD7747 Values"=w1312:string[][])  [unwired: 7 in]
                      n331 = for {
                        tunnel: w1312 -> [w1340] mode=indexing
                        tunnel: [w1341] -> w1311 mode=indexing
                        tunnel: w1313 -> [w1339]
                        tunnel: [w1339] -> w1309
                        n332 = Index Array(array=w1340, index=5) -> (element=w1341:string)
                      }
                    }
                    n333 = local write "STATUS"("VSA Testing...." ("STATUS")) -> ()
                  }
                }
                n334 = Transpose 2D Array(2D array=w1263) -> (transposed array=w1261:string[][])
                n335 = Transpose 2D Array(2D array=w1262) -> (transposed array=w1260:string[][])
                n336 = Transpose 2D Array(2D array=w1259) -> (transposed array=w1258:string[][])
                n337 = Transpose 2D Array(2D array=w1256) -> (transposed array=w1255:string[][])
                n338 = call "WS1050_VSA_Convert_Data.vi"("VSA_C3"=w1255, "error in (no error)"=w1257, "VSA_C2"=w1258, "VSA_C1"=w1260, "Voltage"=w1261) -> ("error out"=w1254:errorcluster, "VSA_V3"=w1251:string[][], "VSA_V2"=w1252:string[][], "VSA_V1"=w1253:string[][])  [unwired: 3 in]
                "VSA_V1" <- w1253
                "VSA_V2" <- w1252
                "VSA_V3" <- w1251
                n339 = case shown="True" w1246 {
                  tunnel: w1273 -> [w1287 w1293]
                  tunnel: [w1287 w1292] -> w1272
                  tunnel: w1254 -> [w1286 w1291]
                  tunnel: [w1286 w1288] -> w1271
                  frame False {
                  }
                  frame True {
                    w1289 = u16 0 items=["Voltage", "Current"] ("Source Mode  (0: Voltage)")
                    n340 = call "Ke2400 Configure Output.vi"("Source Mode  (0: Voltage)"=w1289, "error in (no error)"=w1291, "Output Level (0)"=0.0, "VISA resource name"=w1293) -> ("error out"=w1288:errorcluster, "VISA resource name out"=w1292:refnum<visa-resource-name>)  [unwired: 6 in]
                  }
                }
                n341 = call "Delay.vi"("milliseconds to wait"=u32 50, "error in (no error)"=w1271) -> ("error out"=w1270:errorcluster)  [unwired: 9 in]
              }
              frame #6 {
                # "Handshake Check and EFuse Readback"
                n342 = Or(x=w1361, y=w1366) -> (x .or. y?=w1352:bool)
                n343 = case shown="True" w1352 {
                  tunnel: w1388 -> [w1401 _]
                  tunnel: w1387 -> [w1400 w1406]
                  tunnel: [w1399 w1406] -> w1386
                  tunnel: w1385 -> [w1398 _]
                  tunnel: w1384 -> [w1397 _]
                  tunnel: w1383 -> [w1396 _]
                  tunnel: [w1392 w1405] -> w1382
                  tunnel: [w1391 w1405] -> w1377
                  tunnel: w1353 -> [w1390 _]
                  tunnel: w1371 -> [w1389 _]
                  frame False {
                    n344 = call "WS1050_36DUT_Handshake Check R1_Record All Regs Ver1.0.vi"("file path (use dialog)"=w1401, "Reg1_Bit Cntrl"="Reg1_Bit Cntrl", "File Name"=w1389, "SN"=w1396, "Loop"=w1390, "error"=w1400, "Lot #"=w1398, "Wafer #"=w1397) -> ("Pass/Fail"=→"EFuse Readback Status":bool[], "EFuse Read back"=w1391:string[], "Status"=w1392:string[], "error out"=w1399:errorcluster)  [unwired: 6 in, 2 out]
                    n345 = case shown="0" w1390 {
                      tunnel: w1391 -> [w1402 w1403]
                      frame 0 {
                        "EFuse RB T0" <- w1402
                      }
                      frame 1, Default {
                        "Current EFuse Read back" <- w1403
                      }
                    }
                    n346 = local write "STATUS"("Hand Shake & EFuse Readback...." ("STATUS")) -> ()
                  }
                  frame True {
                    n347 = for {
                      N: 36 -> [_]
                      tunnel: ["NA"] -> w1405 mode=indexing
                    }
                  }
                }
                n348 = Build Array(w1375, w1373, w1372) -> (w1374:string[])
              }
              frame #7 {
                # "Save Data"
                n349 = Increment(x=w1419) -> (x+1=w1418:i32)
                n350 = local write "STATUS"("Saving Data...." ("STATUS")) -> ()
                n351 = Multiply(x=w1418, y=36) -> (x*y=w1413:i32)
                n352 = Path To String(path=w1423) -> (string=w1422:string)
                n353 = Bundle("Test Program"=w1449, "Comment"=w1448, "Data Out"=w1429, "Data Out"=w1428, "Data Out"=w1408, w1427, "Data Out"=w1426, "Data Out"=w1425, "Data Out"=w1424, "Freq(Hz)"=w1411, "Board#"=w1409) -> (w1410:T9)  [unwired: 1 in]
                n354 = case shown="True" "Debug" {
                  tunnel: w1413 -> [w1456 w1459]
                  tunnel: [w1456 w1457] -> w1412
                  frame False {
                  }
                  frame True {
                    n355 = Multiply(x=w1459, y="No of Rows\nFrom Spread Sheet") -> (x*y=w1457:i32)
                  }
                }
                n356 = call "WS1050_36 DUT CV Curve SData Ver1.0.vi"("TMN DC\\CAP Data Log File Path"=w1423, "Lot#"=w1451, "VSA_V1"=w1437, "Wafer#"=w1447, "File Name"=w1416, "error in"=w1454, "TP/Comment"=w1410, "EFuse"=w1441, "Data Output C3"=w1431, "Temperature"=w1435, "VSA_V2"=w1438, "VPI C3"=w1433, "Data Output C1"=w1444, "VPI C2"=w1432, "SN"=w1452, "R/W Status"=w1450, "Cap Header"=w1434, "HD/Cycles Completed"=w1440, "Data Output C2"=w1430, "VSA_V3"=w1436, "Current"=w1443, "VPI C1"=w1442) -> ("error out"=w1453:errorcluster)  [unwired: 5 in]
                n357 = Concatenate Strings(w1422, "\\" ("string"), w1416, "_Multi Socket Data.csv" ("string")) -> (w1421:string)
              }
              frame #8 {
                n358 = case shown="True" "Plot Delta Cmin" {
                  tunnel: w1467 -> [w1483 w1501]
                  tunnel: [w1483 w1497] -> w1461
                  tunnel: w1466 -> [_ w1493]
                  tunnel: w1464 -> [_ w1487]
                  frame False {
                  }
                  frame True {
                    n359 = String To Path(string=w1493) -> (path=w1492:path)
                    n360 = call "Delay.vi"("milliseconds to wait"=u32 50, "error in (no error)"=w1501) -> ("error out"=w1500:errorcluster)  [unwired: 9 in]
                    n361 = call "36DUT Plot From Spread Sheet Updated.vi"("Col C2"="Col C2", "Col C3"="Col C3", "Plot"="Plot", "No of Rows"=w1487, "error in (no error)"=w1500, "Col C1"="Col C1", "Bank"="Bank 1", "file path (dialog if empty)"=w1492) -> ("error out"=w1495:errorcluster, "Delta C_Min Plot"=→"DeltaC Change_1":dbl[][])  [unwired: 2 in]
                    n362 = call "36DUT Plot From Spread Sheet Updated.vi"("Col C2"="Col C2", "Col C3"="Col C3", "Plot"="Plot", "No of Rows"=w1487, "error in (no error)"=w1495, "Col C1"="Col C1", "Bank"="Bank 2", "file path (dialog if empty)"=w1492) -> ("error out"=w1496:errorcluster, "Delta C_Min Plot"=→"DeltaC Change_2":dbl[][])  [unwired: 2 in]
                    n363 = call "36DUT Plot From Spread Sheet Updated.vi"("Col C2"="Col C2", "Col C3"="Col C3", "Plot"="Plot", "No of Rows"=w1487, "error in (no error)"=w1496, "Col C1"="Col C1", "Bank"="Bank 3", "file path (dialog if empty)"=w1492) -> ("error out"=w1497:errorcluster, "Delta C_Min Plot"=→"DeltaC Change_3":dbl[][])  [unwired: 2 in]
                  }
                }
                n364 = Get Date/Time In Seconds() -> (seconds since 1Jan1904=w1470:timestamp)
                n365 = Get Date/Time String(seconds (now)=w1470, want seconds? (F)=TRUE) -> (date string=→"date string":string, time string=→"Previous Time":string)  [unwired: 1 in]
                n366 = Greater Or Equal?(x=w1463, y="TTF Completed") -> (x >= y?=w1462:bool)
                n367 = case shown="True" w1462 {
                  tunnel: w1461 -> [w1476 w1478]
                  tunnel: [w1476 w1477] -> w1460
                  frame False {
                  }
                  frame True {
                    n368 = call "Delay.vi"("milliseconds to wait"=u32 50, "error in (no error)"=w1478) -> ("error out"=w1481:errorcluster)  [unwired: 9 in]
                    n369 = call "WSVCAP SHL Host TL RFFE Write - Multiple DUTs - Common Data.vi"("Data Out"="070201000000", "error in"=w1481, "Log (T)"=FALSE) -> ("error out"=w1477:errorcluster)  [unwired: 12 in]
                  }
                }
                "Loop Completed" <- w1463
              }
            }
            n370 = Compound Arithmetic op=OR(w503, w526) -> (w532:bool)
            n371 = call "Delay.vi"("milliseconds to wait"=u32 10, "error in (no error)"=w435) -> ("error out"=w436:errorcluster)  [unwired: 9 in]
          }
          n372 = Unbundle By Name(w372) -> ("status"=w378:bool)
          n373 = Compound Arithmetic op=OR(w378, w377, w376) -> (w368:bool)
        }
        n374 = for {
          tunnel: w257 -> [w1513]
          tunnel: w238 -> [w1512]
          tunnel: w283 -> [w1510] mode=indexing
          tunnel: [w1505] -> w255
          tunnel: [w1509] -> w282
          n375 = call "E3631A_Voltage Controller updated.vi"("VISA resource name"=w1512, "I_VDD(A)"=0.5, "Channel Controller"=w1510, "Voltage 1"=0.0, "Voltage 2"=3.3, "error in (no error)"=w1513, "I_3.3V (A)"=0.5) -> ("VISA resource name out"=w1509:refnum<visa-resource-name>, "error out"=w1506:errorcluster)  [unwired: 7 in]
          n376 = call "Delay.vi"("milliseconds to wait"=u32 100, "error in (no error)"=w1506) -> ("error out"=w1505:errorcluster)  [unwired: 9 in]
        }
        n377 = VISA Write(VISA resource name=w273, write buffer="SOUR:FUNC VOLT;VOLT:MODE FIX;RANG 100;LEV 0.0;:SENS:FUNC \"CURR\";CURR:PROT 60E-3;RANG 100E-3;:OUTP ON", error in (no error)=w257) -> (VISA resource name out=w271:refnum<visa-resource-name>, error out=w256:errorcluster)  [unwired: 1 out]
        n378 = Merge Errors(w255, w256) -> (w272:errorcluster)
      }
      frame True {
      }
    }
    n379 = Wait Until Next ms Multiple(millisecond multiple=u32 100) -> ()  [unwired: 1 out]
    n380 = Unbundle By Name(w64) -> ("status"=w81:bool)
    n381 = Or(x=w81, y=w73) -> (x .or. y?=w80:bool)
    "STATUS" <- "Idle...." ("STATUS")
  }
  "Ke2000 Out" <- w21
  "PS1 Out" <- w20
  n382 = local write "stop"(w7) -> ()
  n383 = case shown="True" w18 {
    tunnel: [w1530 w1533] -> w2
    tunnel: w12 -> [w1530 w1532]
    frame False {
    }
    frame True {
      n384 = local write "Online"(FALSE ("Online")) -> ()
      n385 = call "WSVCAP SHL Host TL Close.vi"("error in"=w1532) -> ("error out"=w1533:errorcluster)  [unwired: 14 in]
    }
  }
  "error out" <- w2
  n386 = VISA Write(VISA resource name=w13, write buffer="SOUR:FUNC VOLT;VOLT:MODE FIX;RANG 100;LEV 0.0;:SENS:FUNC \"CURR\";CURR:PROT 60E-3;RANG 100E-3;:OUTP OFF", error in (no error)=w12) -> (VISA resource name out=→"VISA resource name out":refnum<visa-resource-name>, error out=→"error out 2":errorcluster)  [unwired: 1 out]
